vi "GUI_Beampointing2.vi"() -> ()   [LabVIEW 2011]
uses:
  GUI_Template/GUI_master/tcp_new_data_event.ctl
  GUI_Template/GUI_master/tcp new data cluster.ctl
  Device Driver/TRAServer/StatusTRA_TypDef.ctl
  Ctrs/beam detection.ctl
  Ctrs/move.ctl
  Ctrs/stats.ctl
  <vilib>/Analysis/NI_AALBase.lvlib
  Device Driver/TRAServer/TRAServer.lvclass
panel:
  in  "Set Centriod Target":bool
  in  "size":dbl=68.1
  in  "Tab Control 2":enum32{"CCD Original ", "CCD Detected"}(tab)=enum."CCD Detected"
  out "image::1":T1(plugin-control) caption="StagingM1Far"
  out "Beam":T1(plugin-control)
  in  "Reset History":bool
  out "centriod X":dbl[](graph)=[269.2727355957031, 269.2727355957031, 269.3190002441406]
  out "centriod Y":dbl[](graph)=[287.58294677734375, 287.58294677734375, 287.771484375]
  out "Stats":cluster{timestamp[], dbl[]}[](graph)
  out "move.Stepsize 2":dbl
  out "move.Stepsize":dbl
  in  "Tab Control":enum32{"System", "Detection", "Feedback"}(tab)=enum."Detection"
  in  "Save Stats":bool
  in  "update speed [ms]":i32=100
  in  "img to avg":i32=5
  in  "Save Config":bool
  in  "Load Config":bool
  in  "UDP Error Message":string
  in  "Cameras":u16(ring)=15 items=["10TW_Driver_Spot_Cam", "B1_TelInput", "B5_CompOut", "B6_SwitchYNear", "GIGEtest", "L7_TREXPass4", "L8_M10Leak", "OAPtestCam", "PaperCam", "StagingAlignBeam1", "StagingAlignBeam2", "StagingCapAlignment", "StagingCapSpec", "StagingCapSpec1stOrder", "StagingChromaxGuppy", "StagingDiodeMonitor", "StagingFocusBeam1", "StagingFocusBeam2", "StagingGuppy", "StagingM1Far", "StagingM1Near", "StagingM3Far", "StagingM4", "StagingM5", "StagingMagnetCam1", "StagingMagnetCam2", "StagingMagnetCam3", "StagingManta2", "StagingModeImager2", "StagingModeTemp", "StagingOAP1Far", "StagingOAP1Near", "StagingOAP2Far", "StagingOAP2Near", "StagingPhasics", "StagingPhosphor", "StagingTapeCam", "StagingTapeMonitorCam", "TREXVarianCam0", "TREXVarianCam1", "TREXVarianCam2", "TREXVarianCam3", "TREX_CapSideView", "TREX_TA6", "TS-253a_in", "TS-CapSideview", "TS-CapSpec", "TS-ChromexCam", "TS-InputNearField", "TS-Mode1", "TS-OverlapCam", "TS-Periscope", "XUV_Cam1", "XUV_Cam2"]
  in  "beam detection para":T2={"Filter"=1, "Filter Para"={"X Size"=5, "Y Size"=5, "% Tolerance"=1}, "detection method"=4, "smal para"=[{"Measurement Parameter"=35, "Range Lower Value"=0.0, "Range Upper Value"=500.0, "Range"=TRUE, "Measurement Type"=FALSE}], "Remove small Objects"=TRUE, "Restrict to round Objects"=TRUE} {"smal para"."Measurement Parameter" items=["Center of Mass X", "Center of Mass Y", "First Pixel X", "First Pixel Y", "Bounding Rect Left", "Bounding Rect Top", "Bounding Rect Right", "Bounding Rect Bottom", "Max Feret Diameter Start X", "Max Feret Diameter Start Y", "Max Feret Diameter End X", "Max Feret Diameter End Y", "Max Horiz. Segment Length Left", "Max Horiz. Segment Length Right", "Max Horiz. Segment Length Row", "-", "Bounding Rect Width", "Bounding Rect Height", "Bounding Rect Diagonal", "Perimeter", "Convex Hull Perimeter", "Holes' Perimeter", "Max Feret Diameter", "Equivalent Ellipse Major Axis", "Equivalent Ellipse Minor Axis", "Equivalent Ellipse Minor Axis (Feret)", "Equivalent Rect Long Side", "Equivalent Rect Short Side", "Equivalent Rect Diagonal", "Equivalent Rect Short Side (Feret)", "Average Horiz. Segment Length", "Average Vert. Segment Length", "Hydraulic Radius", "Waddel Disk Diameter", "-", "Area", "Holes' Area", "Particle & Holes' Area", "Convex Hull Area", "Image Area", "-", "Number of Holes", "Number of Horiz. Segments", "Number of Vert. Segments", "-", "Orientation", "Max Feret Diameter Orientation", "-", "% Area/Image Area", "% Area/(Particle & Holes' Area)", "Ratio of Equivalent Ellipse Axes", "Ratio of Equivalent Rect Sides", "-", "Elongation Factor", "Compactness Factor", "Heywood Circularity Factor", "Type Factor", "-", "Sum X", "Sum Y", "Sum XX", "Sum XY", "Sum YY", "Sum XXX", "Sum XXY", "Sum XYY", "Sum YYY", "-", "Moment of Inertia XX", "Moment of Inertia XY", "Moment of Inertia YY", "Moment of Inertia XXX", "Moment of Inertia XXY", "Moment of Inertia XYY", "Moment of Inertia YYY", "Norm. Moment of Inertia XX", "Norm. Moment of Inertia XY", "Norm. Moment of Inertia YY", "Norm. Moment of Inertia XXX", "Norm. Moment of Inertia XXY", "Norm. Moment of Inertia XYY", "Norm. Moment of Inertia YYY", "Hu Moment 1", "Hu Moment 2", "Hu Moment 3", "Hu Moment 4", "Hu Moment 5", "Hu Moment 6", "Hu Moment 7"]; "smal para"."Range Lower Value" format="%.2f"; "smal para"."Range Upper Value" format="%.2f"; "detection method" items=["clustering", "entropy", "metric", "moments", "inter-class variance"]; "Filter" items=["No Filter", "Median Filter", "Low Pass Filter"]}
  in  "Move Properties":T4={"Tolerance [%]"=10.0, "Stepsize"=0.0, "Invert Axis"=FALSE, "Invert Direction X"=FALSE, "Invert Direction Y"=FALSE, "enable feedback"=FALSE} {"Stepsize" format="%#_6p"}
  out "Y Size":dbl=130.0
  out "X Size":dbl=136.2
  out "Particle Reports (Pixels)":T5(array[cluster])=[{"Area"=12832.0, "Number of Holes"=0.0, "Bounding Rect"={"Left"=200.0, "Top"=223.0, "Right"=335.0, "Bottom"=353.0}, "Center of Mass"={"X"=268.7340243142145, "Y"=287.8902743142145}, "Orientation"=19.894021936277838, "Dimensions"={"Width"=135.0, "Height"=130.0}}] {"Orientation" format="%.2f"; "Dimensions"."Height" format="%.2f"; "Dimensions"."Width" format="%.2f"; "Center of Mass"."Y" format="%.2f"; "Center of Mass"."X" format="%.2f"; "Bounding Rect"."Bottom" format="%.2f"; "Bounding Rect"."Right" format="%.2f"; "Bounding Rect"."Top" format="%.2f"; "Bounding Rect"."Left" format="%.2f"; "Number of Holes" format="%.2f"; "Area" format="%.2f"}
  in  "save cluster":T6={"img to avg"=0, "beam detection para"={"Filter"=0, "Filter Para"={"X Size"=0, "Y Size"=0, "% Tolerance"=0}, "detection method"=0, "smal para"=[], "Remove small Objects"=FALSE, "Restrict to round Objects"=TRUE}, "move"={"Tolerance [%]"=0.0, "Stepsize"=0.0, "Invert Axis"=FALSE, "Invert Direction X"=FALSE, "Invert Direction Y"=FALSE, "enable feedback"=FALSE}} {"beam detection para"."smal para"."Measurement Parameter" items=["Center of Mass X", "Center of Mass Y", "First Pixel X", "First Pixel Y", "Bounding Rect Left", "Bounding Rect Top", "Bounding Rect Right", "Bounding Rect Bottom", "Max Feret Diameter Start X", "Max Feret Diameter Start Y", "Max Feret Diameter End X", "Max Feret Diameter End Y", "Max Horiz. Segment Length Left", "Max Horiz. Segment Length Right", "Max Horiz. Segment Length Row", "-", "Bounding Rect Width", "Bounding Rect Height", "Bounding Rect Diagonal", "Perimeter", "Convex Hull Perimeter", "Holes' Perimeter", "Max Feret Diameter", "Equivalent Ellipse Major Axis", "Equivalent Ellipse Minor Axis", "Equivalent Ellipse Minor Axis (Feret)", "Equivalent Rect Long Side", "Equivalent Rect Short Side", "Equivalent Rect Diagonal", "Equivalent Rect Short Side (Feret)", "Average Horiz. Segment Length", "Average Vert. Segment Length", "Hydraulic Radius", "Waddel Disk Diameter", "-", "Area", "Holes' Area", "Particle & Holes' Area", "Convex Hull Area", "Image Area", "-", "Number of Holes", "Number of Horiz. Segments", "Number of Vert. Segments", "-", "Orientation", "Max Feret Diameter Orientation", "-", "% Area/Image Area", "% Area/(Particle & Holes' Area)", "Ratio of Equivalent Ellipse Axes", "Ratio of Equivalent Rect Sides", "-", "Elongation Factor", "Compactness Factor", "Heywood Circularity Factor", "Type Factor", "-", "Sum X", "Sum Y", "Sum XX", "Sum XY", "Sum YY", "Sum XXX", "Sum XXY", "Sum XYY", "Sum YYY", "-", "Moment of Inertia XX", "Moment of Inertia XY", "Moment of Inertia YY", "Moment of Inertia XXX", "Moment of Inertia XXY", "Moment of Inertia XYY", "Moment of Inertia YYY", "Norm. Moment of Inertia XX", "Norm. Moment of Inertia XY", "Norm. Moment of Inertia YY", "Norm. Moment of Inertia XXX", "Norm. Moment of Inertia XXY", "Norm. Moment of Inertia XYY", "Norm. Moment of Inertia YYY", "Hu Moment 1", "Hu Moment 2", "Hu Moment 3", "Hu Moment 4", "Hu Moment 5", "Hu Moment 6", "Hu Moment 7"]; "beam detection para"."smal para"."Range Lower Value" format="%.2f"; "beam detection para"."smal para"."Range Upper Value" format="%.2f"; "beam detection para"."detection method" items=["clustering", "entropy", "metric", "moments", "inter-class variance"]; "beam detection para"."Filter" items=["No Filter", "Median Filter", "Low Pass Filter"]}
  out "move required":bool
  out "moving":bool
  out "Best Rectangle":T7(array[cluster])=[{"Left"=200.0, "Top"=223.0, "Right"=338.0, "Bottom"=353.0}, {"Left"=200.0, "Top"=223.0, "Right"=338.0, "Bottom"=353.0}, {"Left"=205.0, "Top"=224.0, "Right"=338.0, "Bottom"=350.0}, {"Left"=200.0, "Top"=223.0, "Right"=336.0, "Bottom"=355.0}, {"Left"=200.0, "Top"=223.0, "Right"=336.0, "Bottom"=355.0}]
  out "XY Graph":cluster{timestamp[], dbl[]}[](graph)=[{[timestamp(3452404798.8513913 s since 1904-01-01), timestamp(3452404799.6214356 s since 1904-01-01), timestamp(3452404800.2504716 s since 1904-01-01), timestamp(3452404800.877507 s since 1904-01-01), timestamp(3452404801.5115438 s since 1904-01-01), timestamp(3452404802.1385794 s since 1904-01-01), timestamp(3452404802.7796164 s since 1904-01-01), timestamp(3452404803.4086523 s since 1904-01-01), timestamp(3452404804.1166925 s since 1904-01-01), timestamp(3452404804.7627296 s since 1904-01-01), timestamp(3452404805.403766 s since 1904-01-01), timestamp(3452404806.046803 s since 1904-01-01), timestamp(3452404806.8958516 s since 1904-01-01), timestamp(3452404807.531888 s since 1904-01-01), timestamp(3452404808.174925 s since 1904-01-01), timestamp(3452404808.811961 s since 1904-01-01), timestamp(3452404809.4529977 s since 1904-01-01), timestamp(3452404810.0910344 s since 1904-01-01), timestamp(3452404810.732071 s since 1904-01-01), timestamp(3452404811.373108 s since 1904-01-01)], [-3.53924560546875, -4.652754657642788, -5.44743290091867, -5.300940785876151, -4.715238659785825, -6.004101011596333, -4.752166041728003, -5.050226506875958, -4.109178710453193, -4.665509033203136, -5.175085449218727, -5.028265380859352, -4.379766845703102, -4.631829833984398, -4.844409179687489, -4.304394531250011, -4.530322265624989, -4.936749267578136, -4.763983154296852, -4.448400878906227]}, {[timestamp(3452404798.8513913 s since 1904-01-01), timestamp(3452404799.6214356 s since 1904-01-01), timestamp(3452404800.2504716 s since 1904-01-01), timestamp(3452404800.877507 s since 1904-01-01), timestamp(3452404801.5115438 s since 1904-01-01), timestamp(3452404802.1385794 s since 1904-01-01), timestamp(3452404802.7796164 s since 1904-01-01), timestamp(3452404803.4086523 s since 1904-01-01), timestamp(3452404804.1166925 s since 1904-01-01), timestamp(3452404804.7627296 s since 1904-01-01), timestamp(3452404805.403766 s since 1904-01-01), timestamp(3452404806.046803 s since 1904-01-01), timestamp(3452404806.8958516 s since 1904-01-01), timestamp(3452404807.531888 s since 1904-01-01), timestamp(3452404808.174925 s since 1904-01-01), timestamp(3452404808.811961 s since 1904-01-01), timestamp(3452404809.4529977 s since 1904-01-01), timestamp(3452404810.0910344 s since 1904-01-01), timestamp(3452404810.732071 s since 1904-01-01), timestamp(3452404811.373108 s since 1904-01-01)], [1.230804443359375, -0.3328436558336989, 0.6609996983648898, -0.3690822614664171, 0.27569034847687135, -0.11031780080207909, -0.31644478020683664, 0.5764054032015906, 0.6783385802021371, 0.532257080078125, 0.9677673339843977, 0.27269287109373863, 0.38755493164063637, 0.46185302734375, 0.137542724609375, 0.073089599609375, 0.6028076171875227, 0.7097961425781136, 1.0255981445312727, 0.9409057617187386]}]
  out "Y offset":dbl=0.9409057617187386
  out "X offset":dbl=-4.448400878906227
  in  "Target.X::1":dbl=265.0 min=0.0 max=2000.0 format="%#_6f"
  in  "Target.Y::1":dbl=288.0 min=0.0 max=2000.0 format="%#_6f"
  out "mean Y":dbl=287.05909423828126 format="%0.2f"
  out "mean X":dbl=269.4484008789062 format="%0.2f"
  out "beam detected":bool=TRUE
  in  "Status.Axis 2::2":T8=enum."DISABLE" caption="Status.Axis 1::2"
  in  "Status.Axis 1::2":T8=enum."DISABLE"
  in  "Position.Axis 1::2":dbl=1.39334 caption="TREX M20 X" min=0.0 max=6.0 format="%#_6f"
  in  "Position.Axis 2::2":dbl=4.66198 caption="TREX M20 Y" min=0.0 max=7.0 format="%#_6f"
  in  "GUIdevice 2":string="TREX TRA1"
  out "error out":errorcluster
  in  "insert tag":bool=TRUE
  in  "stop":bool=TRUE
  in  "GUIdevice 1":string="PaperCam"
  out "tcp data event":T9
  out "error IO 2":errorcluster
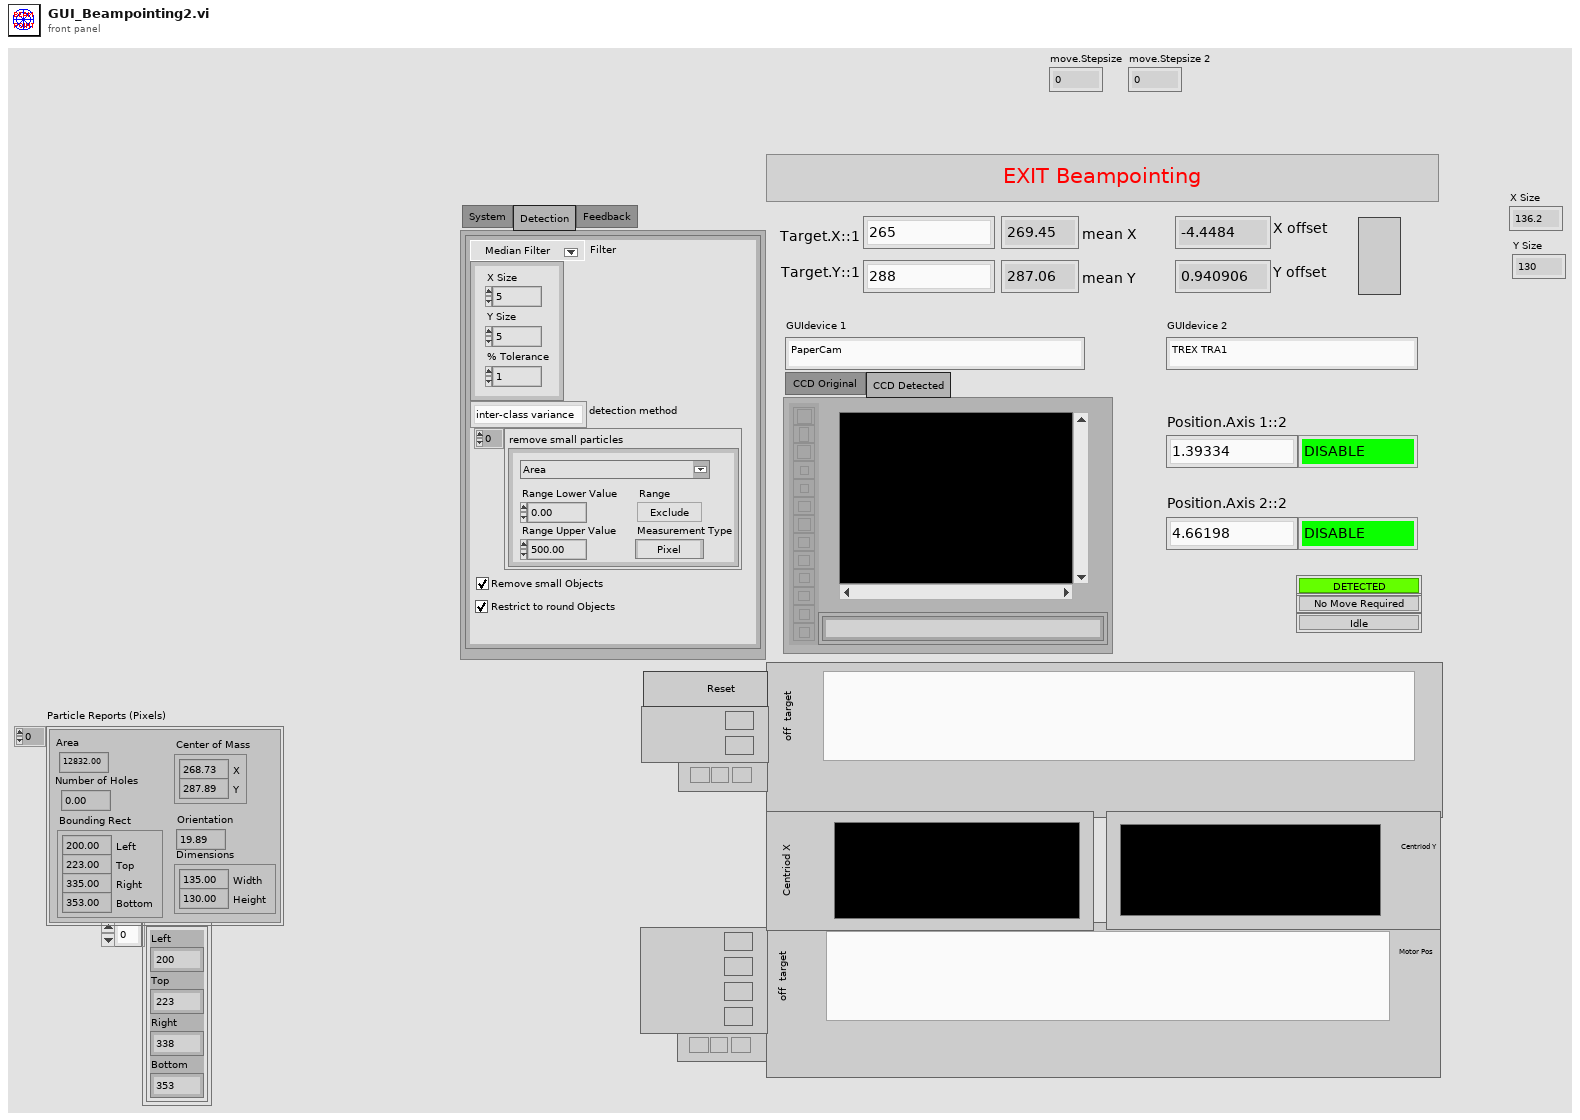
[diagram p1: front panel]
types:
  T1 = typedef "IMAQ Image.ctl" = refnum<image>
  T2 = typedef "beam detection.ctl" = cluster{"Filter":u16, "Filter Para":cluster{"X Size":i32, "Y Size":i32, "% Tolerance":i32}, "detection method":i32, "smal para":cluster{"Measurement Parameter":T3, "Range Lower Value":dbl, "Range Upper Value":dbl, "Range":bool, "Measurement Type":bool}[], "Remove small Objects":bool, "Restrict to round Objects":bool}
  T3 = typedef "Particle Parameters" = i32
  T4 = typedef "move.ctl" = cluster{"Tolerance [%]":dbl, "Stepsize":dbl, "Invert Axis":bool, "Invert Direction X":bool, "Invert Direction Y":bool, "enable feedback":bool}
  T5 = cluster{"Area":dbl, "Number of Holes":dbl, "Bounding Rect":cluster{"Left":dbl, "Top":dbl, "Right":dbl, "Bottom":dbl}, "Center of Mass":cluster{"X":dbl, "Y":dbl}, "Orientation":dbl, "Dimensions":cluster{"Width":dbl, "Height":dbl}}[]
  T6 = cluster{"img to avg":i32, "beam detection para":T2, "move":T4}
  T7 = cluster{"Left":dbl, "Top":dbl, "Right":dbl, "Bottom":dbl}[]
  T8 = typedef "TRAServer.lvclass/StatusTRA_TypDef.ctl" = enum16{"NOT REFERENCED", "CONFIGURATION", "HOMING", "MOVING", "READY", "DISABLE", "JOGGING"}
  T9 = typedef "tcp_new_data_event.ctl" = refnum<user-event>
  T10 = typedef "tcp new data cluster.ctl" = cluster{"EventEnum":enum16{"new data", "connection status update"}, "Device name":string}
  T11 = typedef "Image Type" = u32
  T12 = cluster{"Left":i32, "Top":i32, "Right":i32, "Bottom":i32}
  T13 = enum32{"invalid app kind", "Development System", "Run Time System", "Student Edition", "Embedded LabVIEW", "Evaluation", "Custom"}
  T14 = enum32{"Invalid", "Standard", "Closed", "Hidden", "Minimized", "Maximized"}
  T15 = enum16{"open", "replace", "create", "open or create", "replace or create", "replace or create with confirmation"}
  T16 = typedef "stats.ctl" = cluster{"Stat Centriod X":dbl[], "Stat Centriod Y":dbl[], "TRA Position X":dbl[], "TRA PositionY":dbl[], "Time":timestamp[]}
  T17 = cluster{"Core":cluster{"Current VI Reference":refnum<vi>, "Close Panel on Exit?":bool}, "beam detection para":T2, "Centriod X":dbl[], "Centriod Y":dbl[], "Best Rectangle":cluster{"Left":dbl, "Top":dbl, "Right":dbl, "Bottom":dbl}[], "PArticle Report":cluster{"Area":dbl, "Number of Holes":dbl, "Bounding Rect":cluster{"Left":dbl, "Top":dbl, "Right":dbl, "Bottom":dbl}, "Center of Mass":cluster{"X":dbl, "Y":dbl}, "Orientation":dbl, "Dimensions":cluster{"Width":dbl, "Height":dbl}}[], "Mean Centriod X":dbl[], "Mean Centriod Y":dbl[], "Time":timestamp[], "beam detected":bool, "offsets":cluster{"X offset":dbl, "Y offset":dbl}, "move":T4, "moving":bool, "Stats":T16, "set centriod target":bool}
  T18 = cluster{"Left":dbl, "Top":dbl, "Right":dbl, "Bottom":dbl}
  T19 = cluster{"Current VI Reference":refnum<vi>, "Close Panel on Exit?":bool}
  T20 = cluster{"Time":timestamp[], "Stat Centriod X":dbl[]}
  T21 = cluster{"Time":timestamp[], "Stat Centriod Y":dbl[]}
  T22 = cluster{"Time":timestamp[], "TRA Position X":dbl[]}
  T23 = cluster{"Time":timestamp[], "TRA PositionY":dbl[]}
  T24 = cluster{"Time":timestamp[], "TRA PositionY":dbl[]}[]
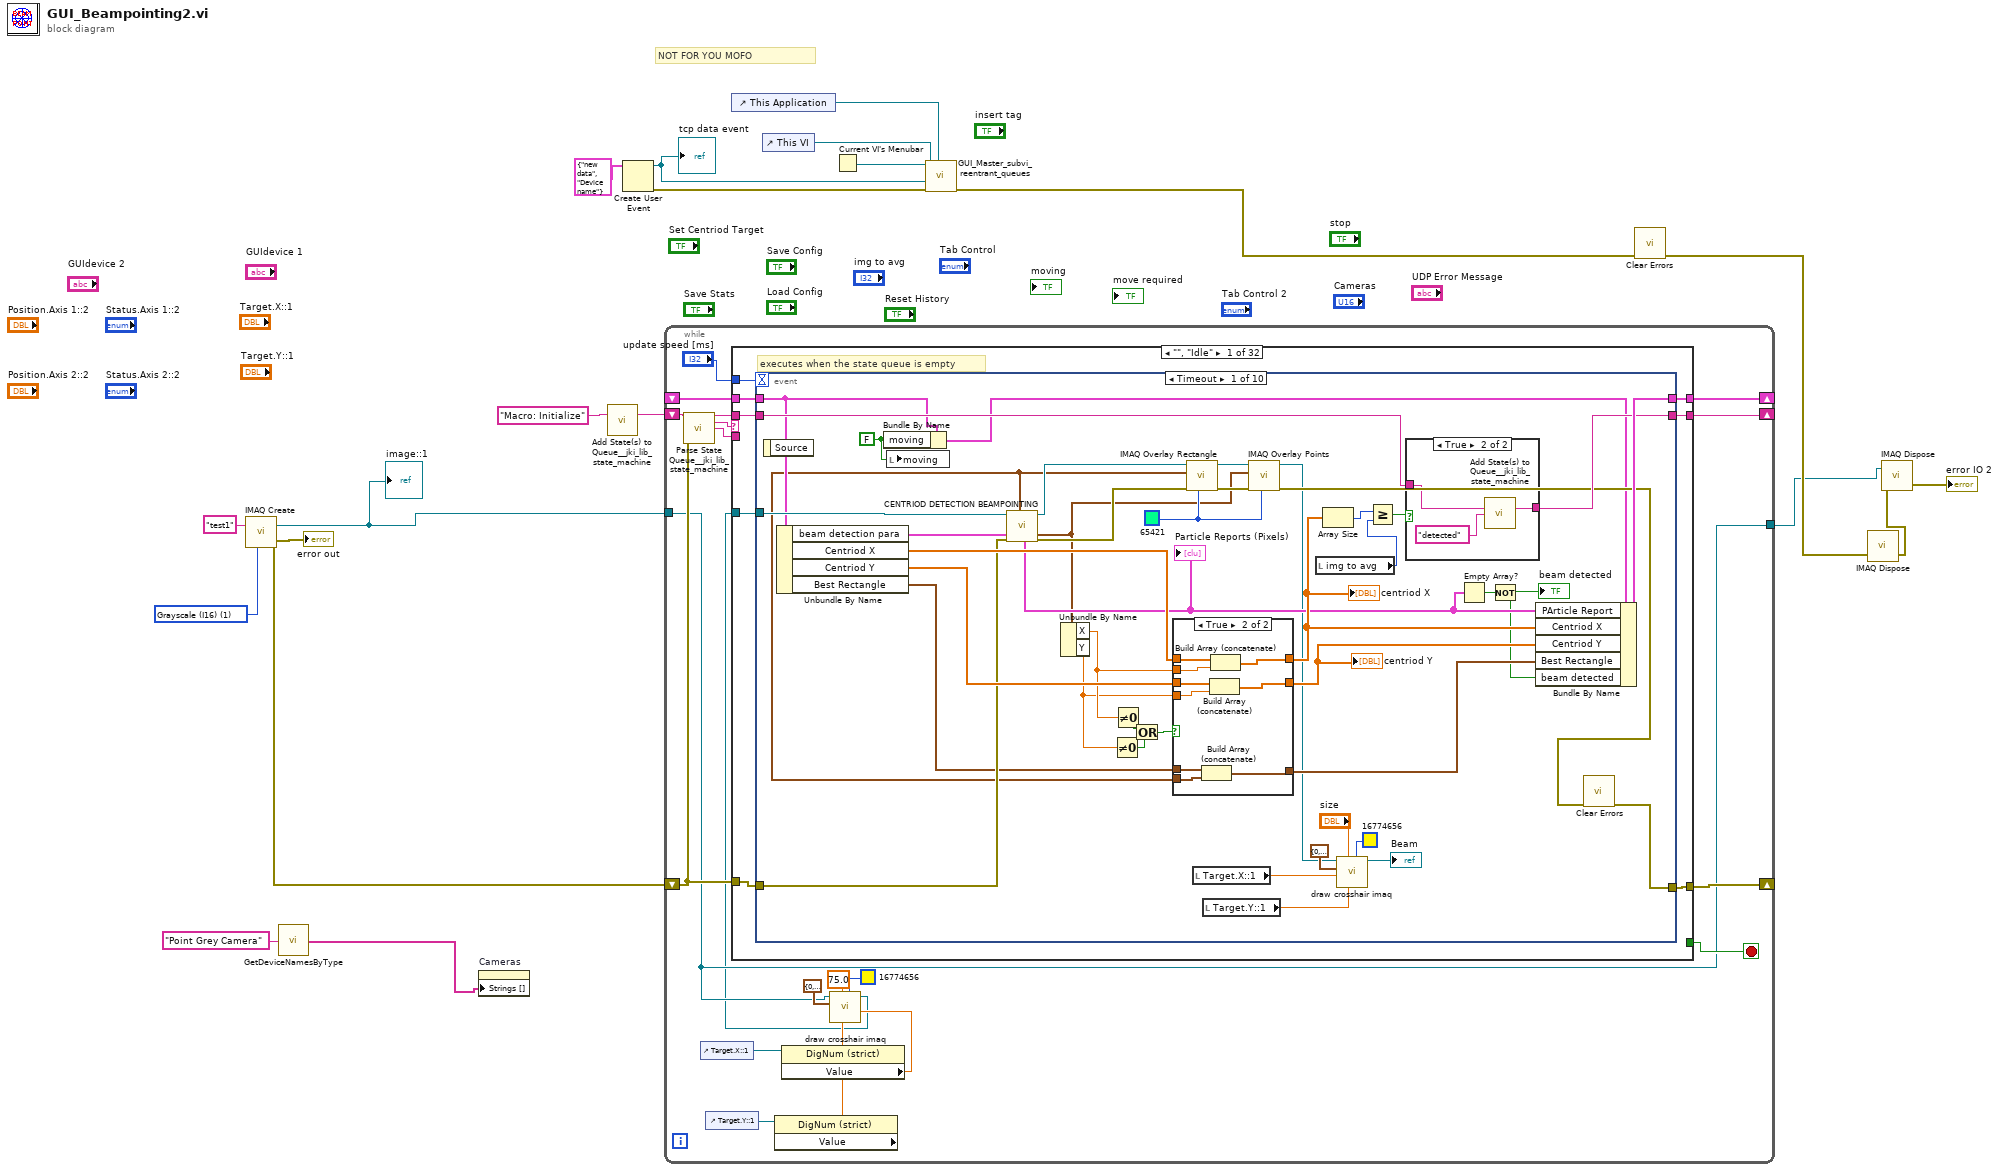
[diagram p0: block diagram]
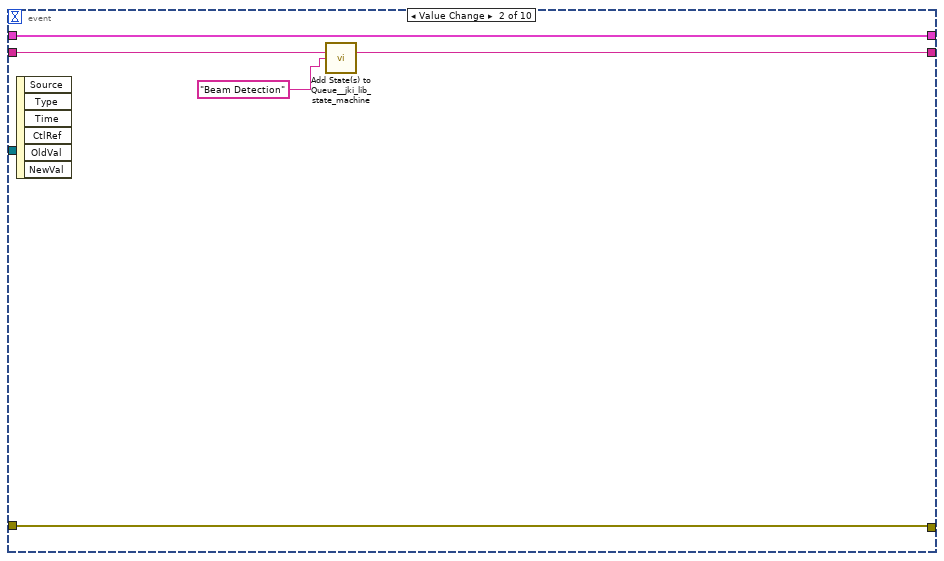
[diagram p4: hidden frame]
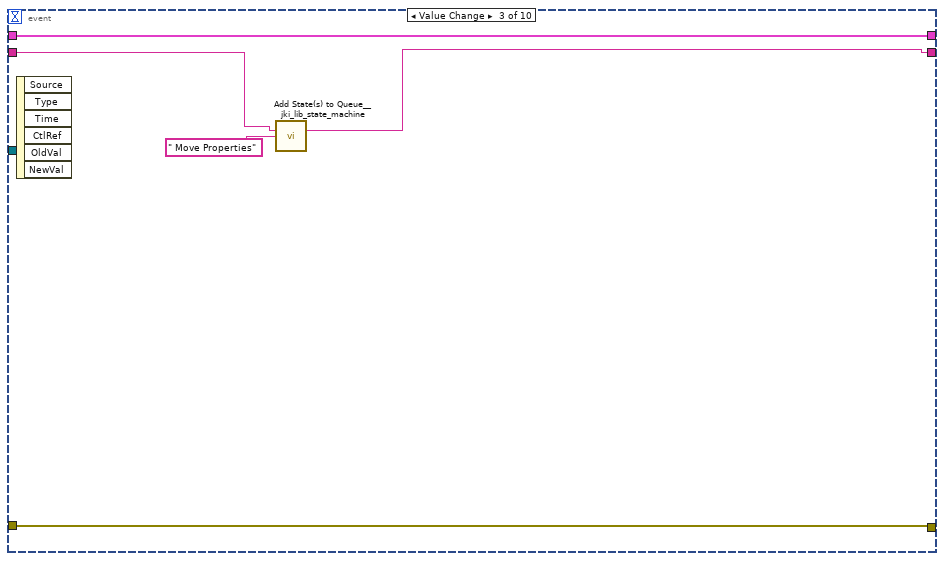
[diagram p5: hidden frame]
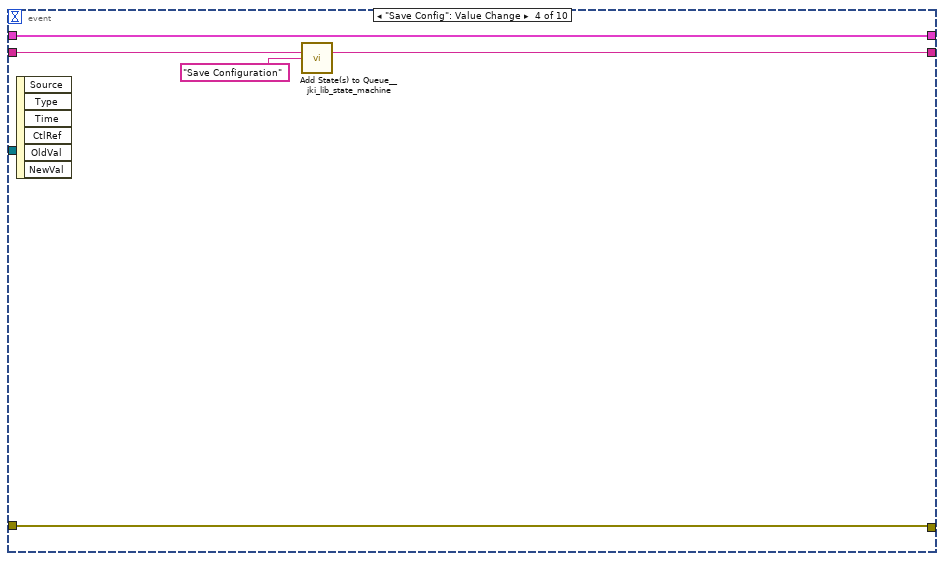
[diagram p6: hidden frame]
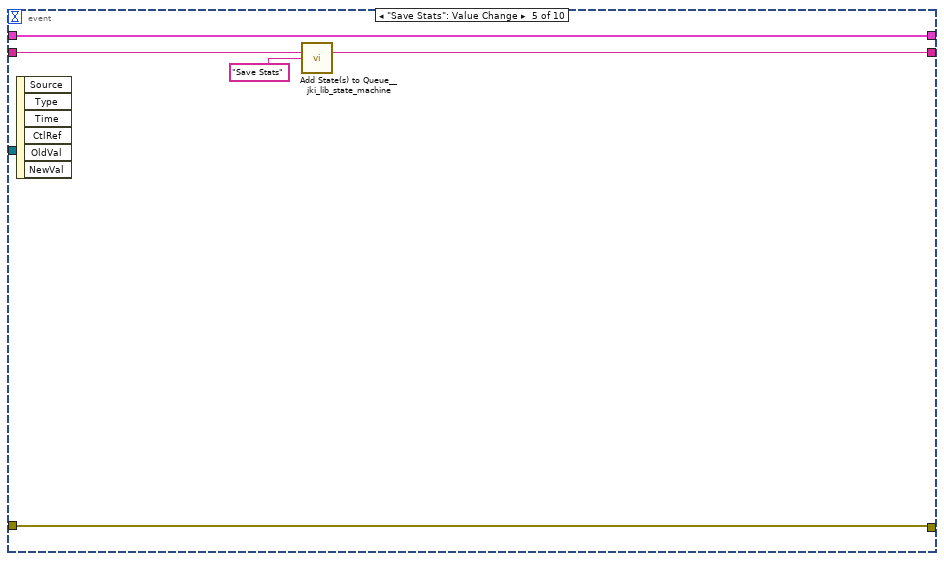
[diagram p7: hidden frame]
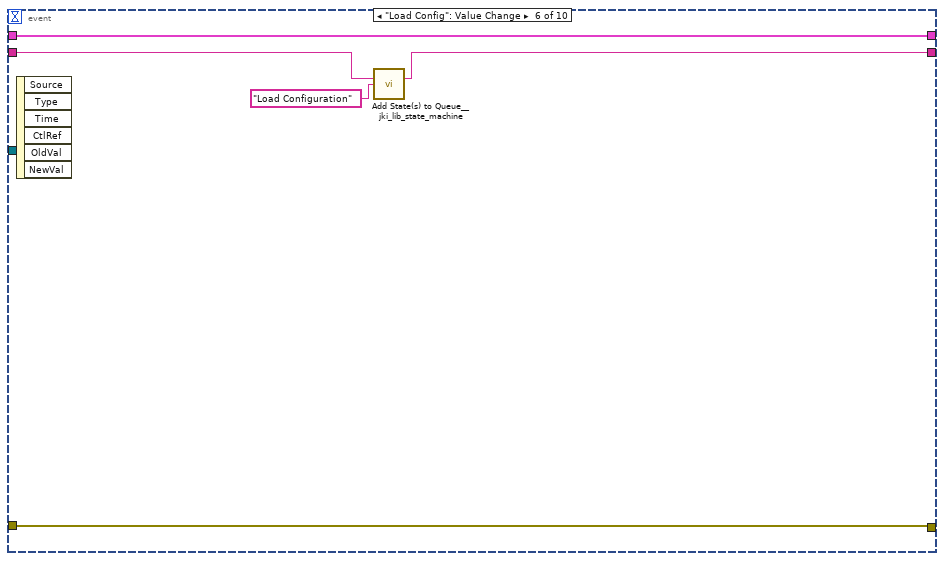
[diagram p8: hidden frame]
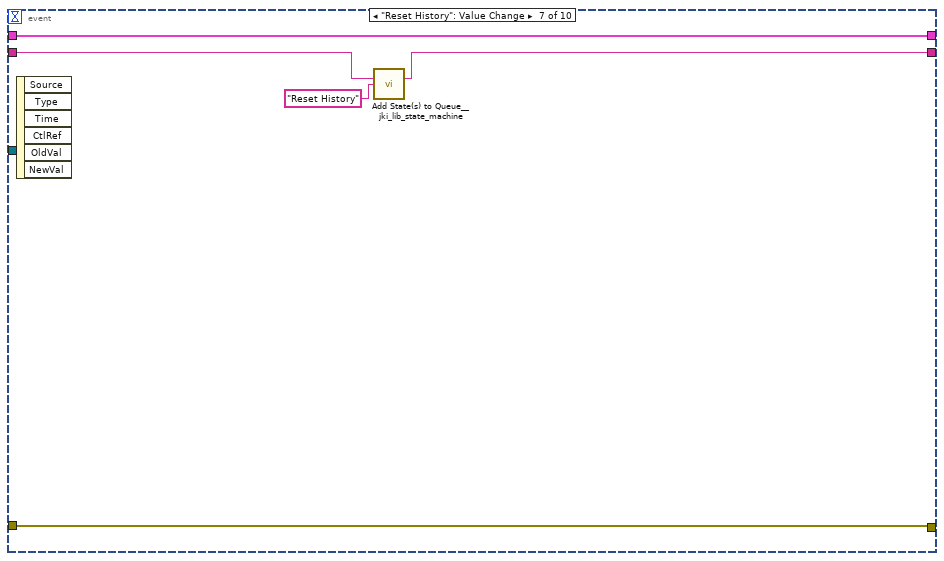
[diagram p9: hidden frame]
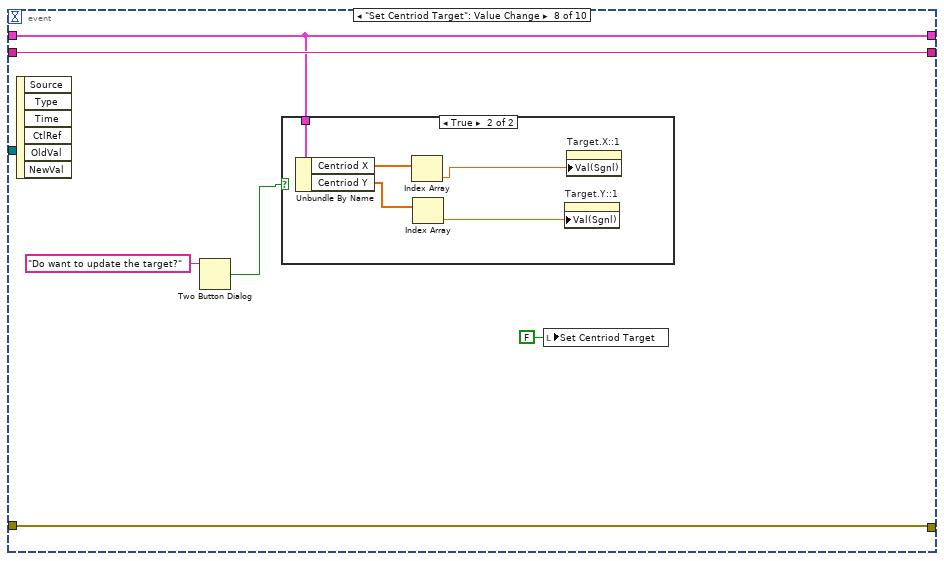
[diagram p10: hidden frame]
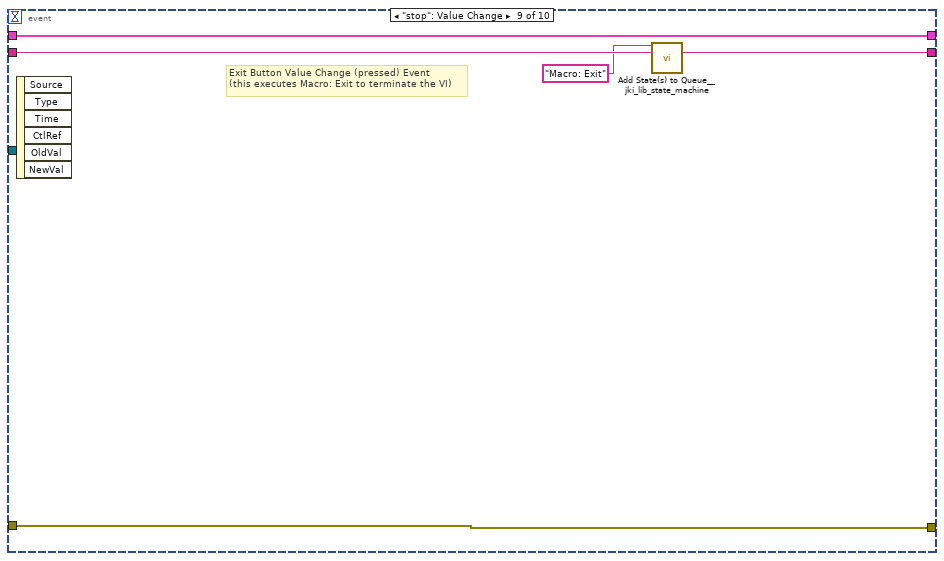
[diagram p12: hidden frame]
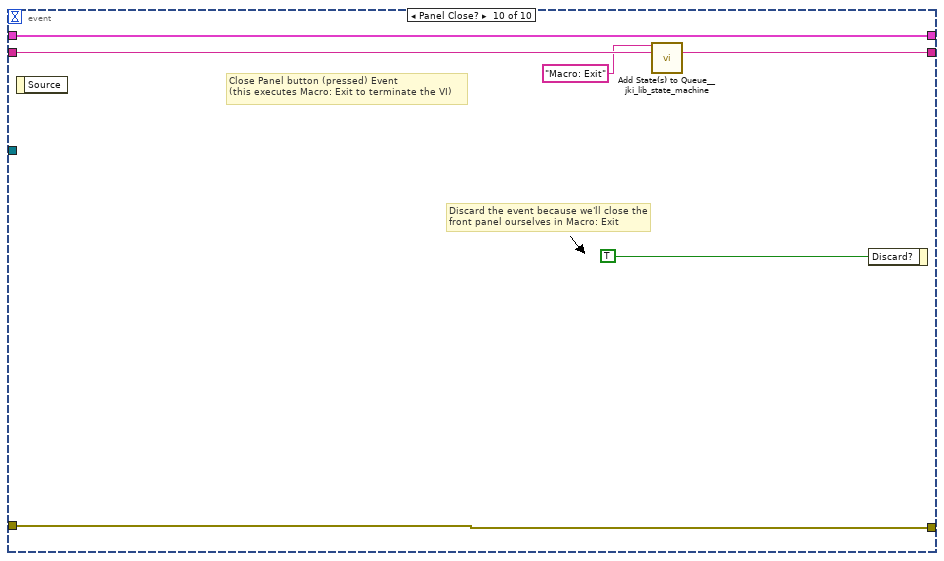
[diagram p13: hidden frame]
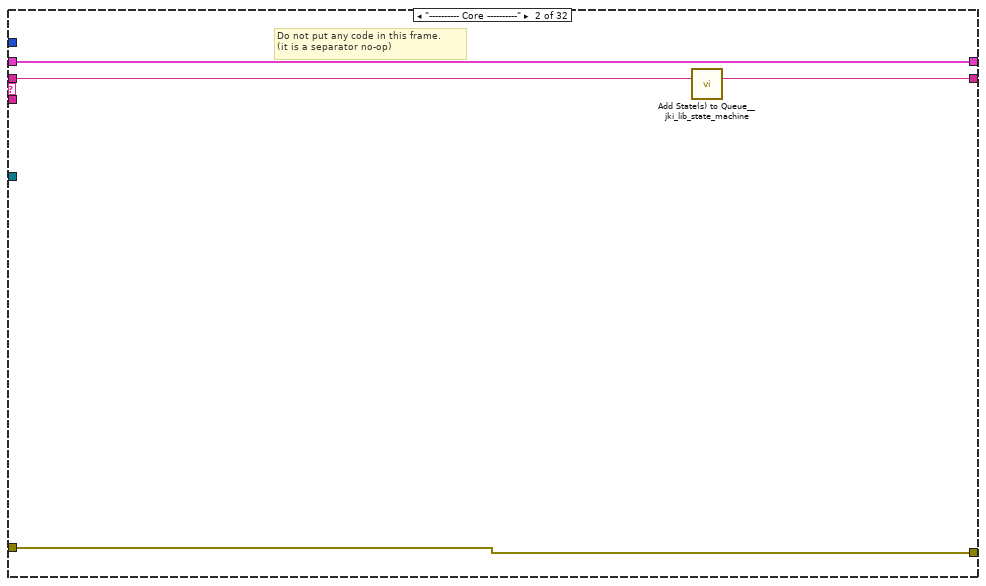
[diagram p14: hidden frame]
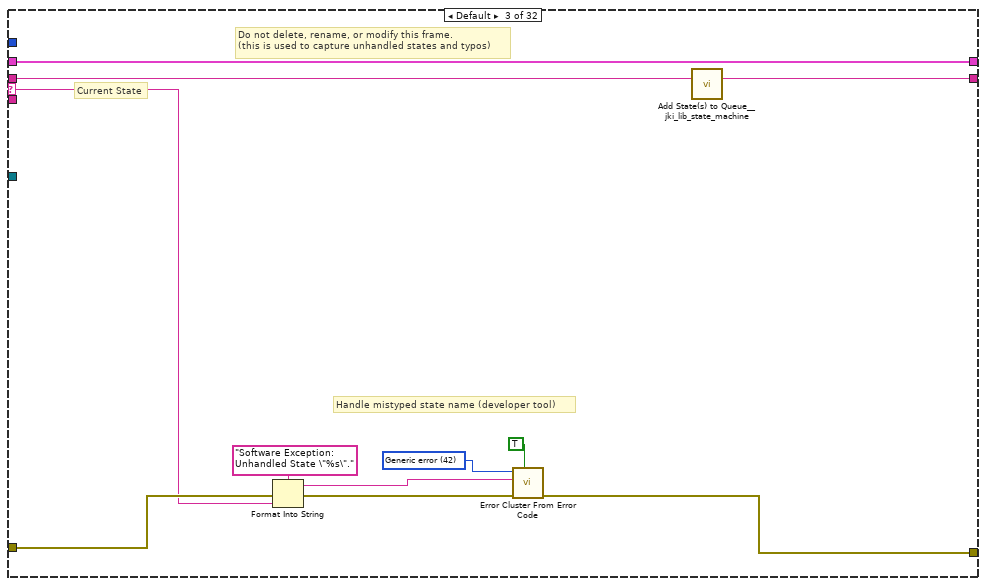
[diagram p15: hidden frame]
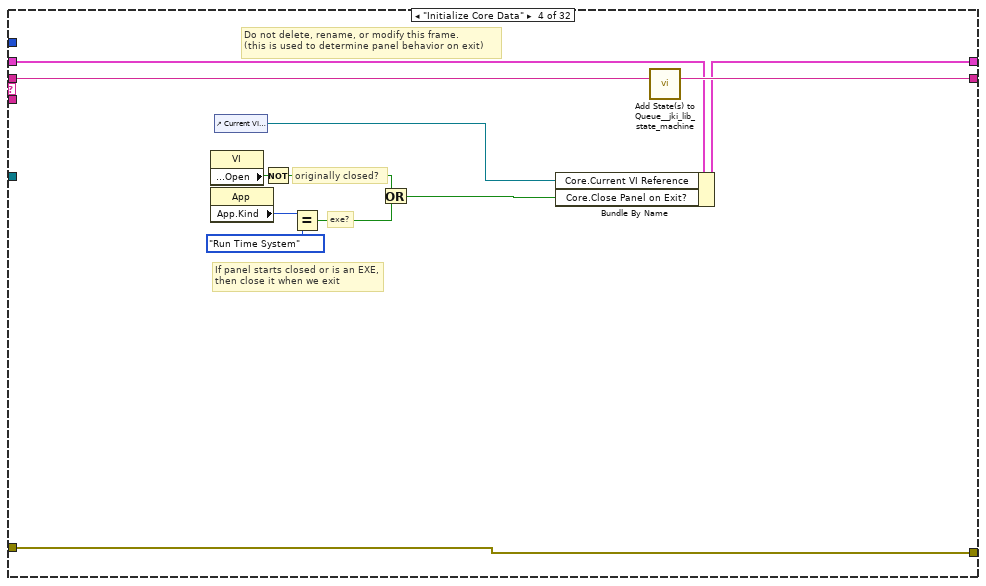
[diagram p16: hidden frame]
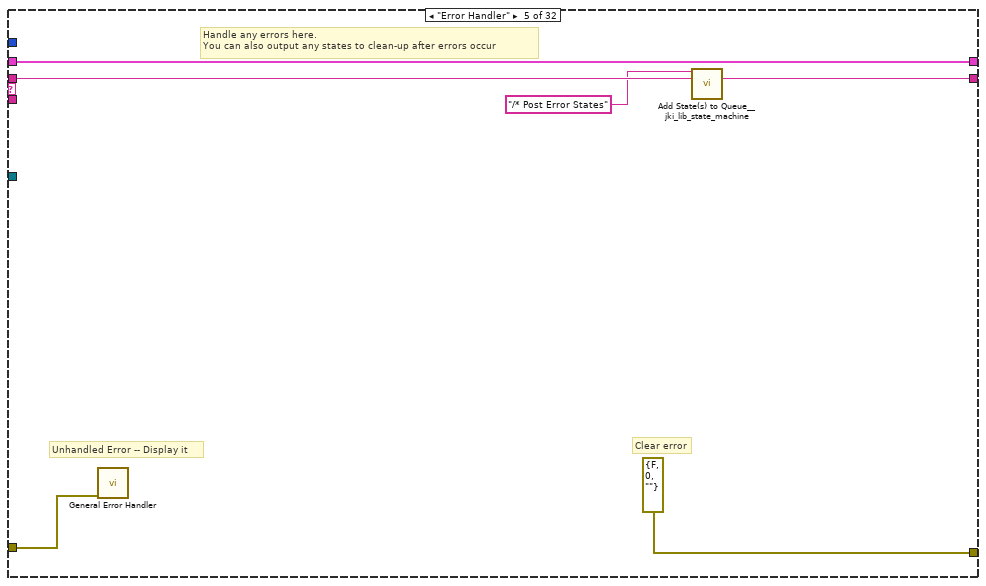
[diagram p17: hidden frame]
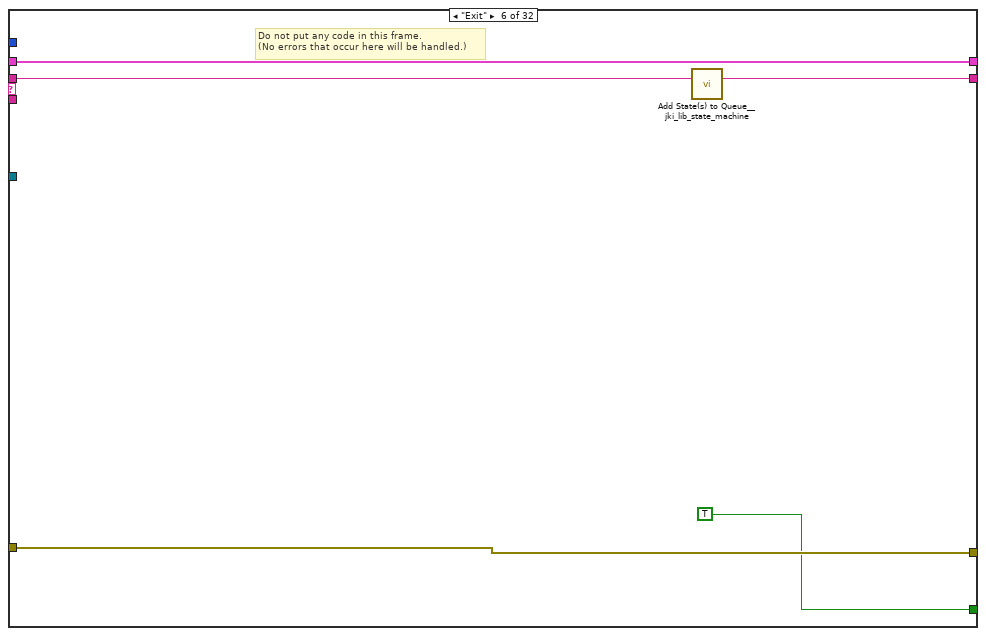
[diagram p18: hidden frame]
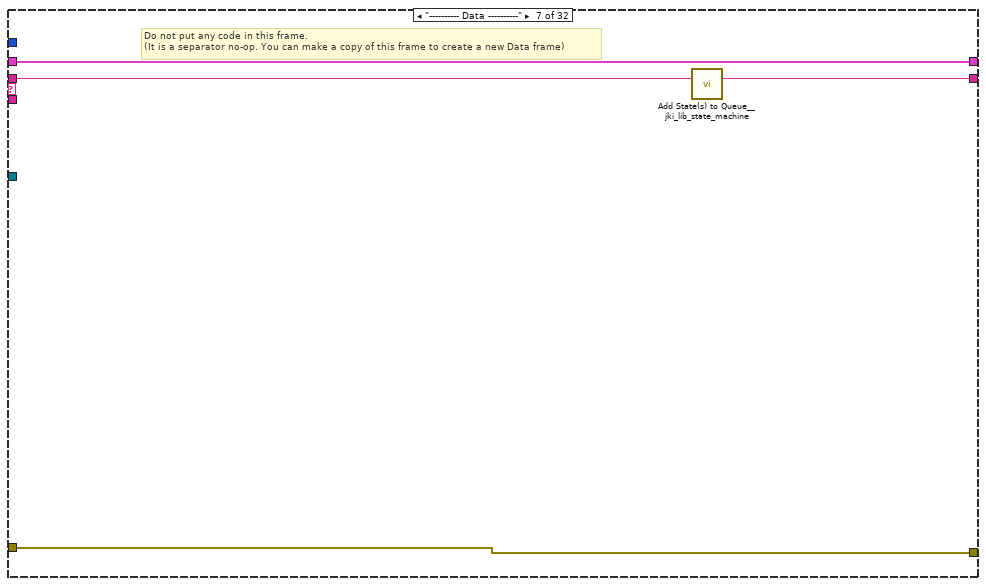
[diagram p19: hidden frame]
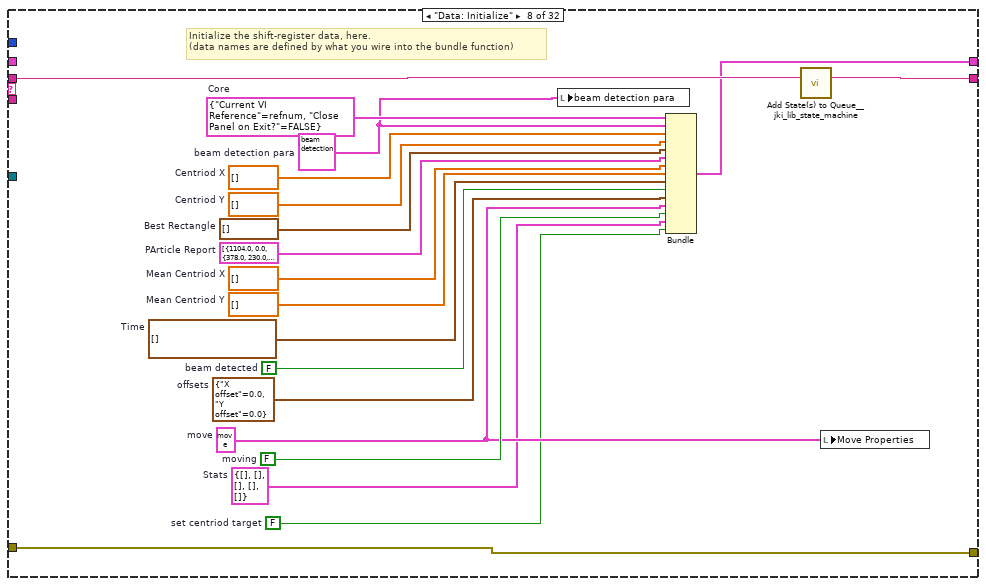
[diagram p20: hidden frame]
diagram:
  w18 = T11 1 items=["Grayscale (U8)", "Grayscale (I16)", "Grayscale (SGL)", "Complex (CSG)", "RGB (U32)", "HSL (U32)", "RGB (U64)", "Grayscale (U16)"] ("Image Type")
  # "NOT FOR YOU MOFO"
  n1 = call "IMAQ Create"("Image Name"="test1", "Image Type"=w18) -> ("New Image"=w3:T1, "error out"=w11:errorcluster)  [unwired: 3 in]
  "error out" <- w11
  "image::1" <- w3
  n2 = call "GetDeviceNamesByType.vi"("Device Type"="Point Grey Camera") -> ("Array"=w1:string[])
  n3 = property on="Cameras" class="Ring (strict)"("Strings []"=w1) -> ()  [unwired: 2 in, 2 out]
  n4 = call <vilib>:"Add State(s) to Queue__jki_lib_state_machine.vi"("State(s) in (\"\")"="Macro: Initialize") -> ("States Out"=w13:string)  [unwired: 14 in]
  n5 = Create User Event(user event datatype=T10 {"EventEnum"=enum."new data", "Device name"="Device name"} ("New Event")) -> (user event=w4:refnum<user-event>, error out=w6:errorcluster)  [unwired: 1 in]
  "tcp data event" <- w4
  n6 = while "JKI - String-Based Queued State Machine (Basic) v1.0" {
    shift-right: [w33] -> _
    shift-left: _ -> [w32]
    shift-right: [w35] -> _
    shift-left: w11 -> [w30]
    shift-right: [w34] -> _
    shift-left: w13 -> [w36]
    tunnel: w3 -> [w21]
    tunnel: [w21] -> w10
    stop <- w29 stop-if-true
    n7 = call <vilib>:"Parse State Queue__jki_lib_state_machine.vi"("State Queue"=w36, "Error In (no error)"=w30) -> ("Remaining States"=w38:string, "Current State"=w39:string, "Arguments"=w37:string)  [unwired: 11 in]
    n8 = control-ref of="Target.X::1"() -> (w25:refnum<vi>)
    n9 = control-ref of="Target.Y::1"() -> (w26:refnum<vi>)
    n10 = property class="DigNum (strict)"(reference=w26) -> ("Value"=w28:dbl)  [unwired: 1 in, 2 out]
    n11 = property class="DigNum (strict)"(reference=w25) -> ("Value"=w27:dbl)  [unwired: 1 in, 2 out]
    n12 = call "draw crosshair imaq.vi"("Color"=u32 16774656, "Target.Y"=w28, "size"=75.0, "Target.X"=w27, "Bounding Rectangle"=T12 {"Left"=0, "Top"=0, "Right"=0, "Bottom"=0}, "image in"=w21) -> ("image out"=w20:T1)  [unwired: 5 in]
    n13 = case shown="\"\", \"Idle\"" w39 {
      selector: w39 -> [_ _ w162 _ _ _ _ _ _ _ _ _ _ _ _ _ _ _ _ _ _ _ _ _ _ _ _ _ _ _ _ _]
      tunnel: w38 -> [w47 w161 w166 w184 w190 w195 w199 w218 w224 w228 w232 w238 w249 w275 w280 w290 w294 w300 w306 w321 w333 w349 w356 w360 w387 w393 w430 w443 w488 w528 w565 w569]
      tunnel: w37 -> [_ _ _ _ _ _ _ _ _ _ _ w233 w243 _ _ _ _ _ _ _ _ _ _ _ _ _ _ _ _ _ _ _]
      tunnel: w32 -> [w45 w158 w164 w175 w187 w193 w196 _ w220 w225 w230 w236 w245 w272 w277 w287 w291 w296 w302 w317 w329 w340 w352 w357 w367 w395 w427 w433 w479 w525 w557 w566]
      tunnel: [w44 w159 w168 w181 errorcluster {"status"=FALSE, "code"=0, "source"=""} ("error out") w192 w197 w215 w221 w226 w229 w234 w246 w273 w278 w288 w292 w298 w304 w308 w324 w337 w354 w358 w385 w414 w428 w441 w486 w526 w563 w567] -> w35
      tunnel: w30 -> [w43 w159 w167 w181 w186 w192 w197 w215 w222 w226 w229 w235 w247 w273 w278 w288 w292 w298 w304 w309 w325 w338 w354 w358 w385 w414 w428 w441 w486 w526 w563 w567]
      tunnel: [w46 w160 w165 w183 w189 w194 w198 w217 w223 w227 w231 w237 w248 w274 w279 w289 w293 w299 w305 w320 w332 w348 w355 w359 w386 w401 w429 w442 w487 w527 w564 w568] -> w34
      tunnel: [_ _ _ _ _ TRUE _ _ _ _ _ _ _ _ _ _ _ _ _ _ _ _ _ _ _ _ _ _ _ _ _ _] -> w29
      tunnel: [w42 w158 w164 w182 w187 w193 w196 w216 w220 w225 w230 w236 w245 w272 w277 w287 w291 w295 w301 w317 w329 w339 w351 w357 w366 w399 w427 w435 w478 w523 w546 w566] -> w33
      tunnel: "update speed [ms]" -> [w41 _ _ _ _ _ _ _ _ _ _ _ _ _ _ _ _ _ _ _ _ _ _ _ _ _ _ _ _ _ _ _]
      tunnel: w20 -> [w40 _ _ _ _ _ _ _ _ _ _ _ _ _ _ _ _ _ _ _ _ _ _ _ _ _ _ _ _ _ _ _]
      frame "", "Idle" {
        # "executes when the state queue is empty"
        n14 = event shown="[0] Timeout" {
          selector: _ -> [_ _ _ _ _ _ _ _ _ _]
          dyn-events: _ -> [_ _ _ _ _ _ _ _ _ _]
          timeout: w41 -> [_ _ _ _ _ _ _ _ _ _]
          tunnel: w47 -> [w69 w109 w114 w119 w124 w128 w133 w140 w151 w157]
          tunnel: [w68 w108 w112 w117 w122 w127 w132 w140 w150 w156] -> w46
          tunnel: w45 -> [w59 w110 w115 w120 w125 w130 w135 w139 w148 w154]
          tunnel: [w65 w107 w111 w116 w121 w129 w134 w141 w149 w155] -> w44
          tunnel: w43 -> [w84 w107 w111 w116 w121 w129 w134 w141 w149 w155]
          tunnel: [w87 w110 w115 w120 w125 w130 w135 w139 w148 w154] -> w42
          tunnel: w40 -> [w88 _ _ _ _ _ _ _ _ _]
          event Timeout {
            w57 = FALSE ("moving")
            w76 = u32 65421 ("Color")
            n15 = event-data() -> ()  [unwired: 1 in, 1 out]
            n16 = Unbundle By Name(w59) -> ("beam detection para"=w89:T2, "Centriod X"=w86:dbl[], "Centriod Y"=w85:dbl[], "Best Rectangle"=w78:T7)
            n17 = Bundle By Name(cluster=w59, "moving"=w57) -> (w58:T17)
            n18 = local write "moving"(w57) -> ()
            n19 = call "CENTRIOD DETECTION BEAMPOINTING.vi"("Refnum in"=w88, "beam detection para"=w89, "error in (no error)"=w84) -> ("Bounding Rect"=w48:T18, "Particle Reports (Pixels)"=w62:T5, "Refnum out"=w73:T1, "Centriod"=w49:cluster{"X":dbl, "Y":dbl}, "error out"=w67:errorcluster)  [unwired: 10 in, 2 out]
            "Particle Reports (Pixels)" <- w62
            n20 = Unbundle By Name(w49) -> ("X"=w81:dbl, "Y"=w80:dbl)
            n21 = Not Equal To 0?(x=w80) -> (x != 0?=w83:bool)
            n22 = Not Equal To 0?(x=w81) -> (x != 0?=w82:bool)
            n23 = Or(x=w82, y=w83) -> (x .or. y?=w79:bool)
            n24 = case shown="True" w79 {
              tunnel: w86 -> [w96 w105]
              tunnel: w85 -> [w95 w104]
              tunnel: [w96 w103] -> w71
              tunnel: [w95 w102] -> w72
              tunnel: w81 -> [_ w101]
              tunnel: w80 -> [_ w100]
              tunnel: w78 -> [w94 w99]
              tunnel: w48 -> [_ w98]
              tunnel: [w94 w97] -> w77
              frame False {
              }
              frame True {
                n25 = Build Array (concatenate)(w99, w98) -> (w97:T7)
                n26 = Build Array (concatenate)(w104, w100) -> (w102:dbl[])
                n27 = Build Array (concatenate)(w105, w101) -> (w103:dbl[])
              }
            }
            "centriod X" <- w71
            "centriod Y" <- w72
            n28 = call "IMAQ Overlay Rectangle"("Color"=w76, "error in (no error)"=w67, "Rectangle"=w48, "Image"=w73) -> ("error out"=w74:errorcluster, "Image Out"=w75:T1)  [unwired: 6 in]
            n29 = local read "Target.X::1"() -> (w51:dbl)
            n30 = local read "Target.Y::1"() -> (w50:dbl)
            n31 = call "IMAQ Overlay Points"("Color"=w76, "error in (no error)"=w74, "Point"=w49, "Image"=w75) -> ("error out"=w66:errorcluster, "Image Out"=w53:T1)  [unwired: 6 in]
            n32 = local read "img to avg"() -> (w63:i32)
            n33 = Array Size(array=w71) -> (size(s)=w64:i32)
            n34 = call "draw crosshair imaq.vi"("Color"=u32 16774656, "Target.Y"=w50, "size"="size", "Target.X"=w51, "Bounding Rectangle"=T12 {"Left"=0, "Top"=0, "Right"=0, "Bottom"=0}, "image in"=w53) -> ("image out"=→"Beam":T1)  [unwired: 5 in]
            n35 = Greater Or Equal?(x=w64, y=w63) -> (x >= y?=w70:bool)
            n36 = case shown="True" w70 {
              tunnel: w69 -> [w90 w93]
              tunnel: [w90 w92] -> w68
              frame False {
              }
              frame True {
                n37 = call <vilib>:"Add State(s) to Queue__jki_lib_state_machine.vi"("State(s) in (\"\")"=w93, "State(s) at Back (\"\")"="detected" ("State(s) in Front (\"\")")) -> ("States Out"=w92:string)  [unwired: 13 in]
              }
            }
            n38 = Empty Array?(array=w62) -> (empty?=w61:bool)
            n39 = Not(x=w61) -> (.not. x?=w60:bool)
            "beam detected" <- w60
            n40 = Bundle By Name(cluster=w58, "PArticle Report"=w62, "Centriod X"=w71, "Centriod Y"=w72, "Best Rectangle"=w77, "beam detected"=w60) -> (w87:T17)
            n41 = call <vilib>:"Clear Errors.vi"("error in (no error)"=w66) -> ("error out"=w65:errorcluster)  [unwired: 6 in]
          }
          event Value Change {
            n42 = event-data() -> ()  [unwired: 1 in, 6 out]
            n43 = call <vilib>:"Add State(s) to Queue__jki_lib_state_machine.vi"("State(s) in (\"\")"=w109, "State(s) at Back (\"\")"="Beam Detection" ("State(s) at Back (\"\")")) -> ("States Out"=w108:string)  [unwired: 13 in]
          }
          event Value Change {
            n44 = event-data() -> ()  [unwired: 1 in, 6 out]
            n45 = call <vilib>:"Add State(s) to Queue__jki_lib_state_machine.vi"("State(s) in (\"\")"=w114, "State(s) at Back (\"\")"=" Move Properties" ("State(s) at Back (\"\")")) -> ("States Out"=w112:string)  [unwired: 13 in]
          }
          event "Save Config": Value Change {
            n46 = event-data() -> ()  [unwired: 1 in, 6 out]
            n47 = call <vilib>:"Add State(s) to Queue__jki_lib_state_machine.vi"("State(s) in (\"\")"=w119, "State(s) at Back (\"\")"="Save Configuration" ("State(s) in Front (\"\")")) -> ("States Out"=w117:string)  [unwired: 13 in]
          }
          event "Save Stats": Value Change {
            n48 = event-data() -> ()  [unwired: 1 in, 6 out]
            n49 = call <vilib>:"Add State(s) to Queue__jki_lib_state_machine.vi"("State(s) in (\"\")"=w124, "State(s) at Back (\"\")"="Save Stats" ("State(s) in Front (\"\")")) -> ("States Out"=w122:string)  [unwired: 13 in]
          }
          event "Load Config": Value Change {
            n50 = event-data() -> ()  [unwired: 1 in, 6 out]
            n51 = call <vilib>:"Add State(s) to Queue__jki_lib_state_machine.vi"("State(s) in (\"\")"=w128, "State(s) at Back (\"\")"="Load Configuration" ("State(s) in Front (\"\")")) -> ("States Out"=w127:string)  [unwired: 13 in]
          }
          event "Reset History": Value Change {
            n52 = event-data() -> ()  [unwired: 1 in, 6 out]
            n53 = call <vilib>:"Add State(s) to Queue__jki_lib_state_machine.vi"("State(s) in (\"\")"=w133, "State(s) at Back (\"\")"="Reset History" ("State(s) in Front (\"\")")) -> ("States Out"=w132:string)  [unwired: 13 in]
          }
          event "Set Centriod Target": Value Change {
            n54 = event-data() -> ()  [unwired: 1 in, 6 out]
            n55 = Two Button Dialog(message="Do want to update the target?") -> (T button?=w136:bool)  [unwired: 2 in]
            n56 = case shown="True" w136 {
              tunnel: w139 -> [_ w146]
              frame False {
              }
              frame True {
                n57 = Unbundle By Name(w146) -> ("Centriod X"=w145:dbl[], "Centriod Y"=w143:dbl[])
                n58 = Index Array(array=w145) -> (element=w144:dbl)  [unwired: 1 in]
                n59 = Index Array(array=w143) -> (element=w142:dbl)  [unwired: 1 in]
                n60 = property on="Target.Y::1" class="DigNum (strict)"("Val(Sgnl)"=w142) -> ()  [unwired: 2 in, 2 out]
                n61 = property on="Target.X::1" class="DigNum (strict)"("Val(Sgnl)"=w144) -> ()  [unwired: 2 in, 2 out]
              }
            }
            n62 = local write "Set Centriod Target"(FALSE ("Set Centriod Target")) -> ()
          }
          event "stop": Value Change {
            # "Exit Button Value Change (pressed) Event\n(this executes Macro: Exit to terminate the VI)"
            n63 = event-data() -> ()  [unwired: 1 in, 6 out]
            n64 = call <vilib>:"Add State(s) to Queue__jki_lib_state_machine.vi"("State(s) in Front (\"\")"="Macro: Exit", "State(s) in (\"\")"=w151) -> ("States Out"=w150:string)  [unwired: 13 in]
          }
          event Panel Close? {
            # "Discard the event because we'll close the front panel ourselves in Macro: Exit"
            # "Close Panel button (pressed) Event\n(this executes Macro: Exit to terminate the VI)"
            n65 = event-data() -> ()  [unwired: 1 in, 1 out]
            n66 = call <vilib>:"Add State(s) to Queue__jki_lib_state_machine.vi"("State(s) in Front (\"\")"="Macro: Exit", "State(s) in (\"\")"=w157) -> ("States Out"=w156:string)  [unwired: 13 in]
            n67 = event-data("Discard?"=TRUE) -> ()  [unwired: 1 in, 1 out]
          }
        }
      }
      frame "---------- Core ----------" {
        # "Do not put any code in this frame.\n(it is a separator no-op)"
        n68 = call <vilib>:"Add State(s) to Queue__jki_lib_state_machine.vi"("State(s) in (\"\")"=w161) -> ("States Out"=w160:string)  [unwired: 14 in]
      }
      frame Default {
        w171 = 42 items=["No error", "Argument error", "Memory is full", "Out of zone", "End of file", "File already open", "Generic file I/O error", "File not found", "File permission error", "Disk is full", "Duplicate path", "Too many files open", "System feature not enabled", "Resource file not found", "Cannot add resource", "Resource not found", "Image not found", "Image memory error", "Pen does not exist", "Config type invalid", "Config token not found", "Config parse error", "Config memory error", "Bad external code format", "Bad external code offset", "External code not present", "Null window", "Destroy window error", "Null menu", "Print aborted", "Bad print record", "Print driver error", "Windows error during printing", "Memory error during printing", "Print dialog error", "Generic print error", "Invalid device refnum", "Device not found", "Device parameter error", "Device unit error", "Cannot open device", "Device call aborted", "Generic error", "Cancelled by user", "Object ID too low", "Object ID too high", "Object not in heap", "Unknown heap", "Unknown object (invalid DefProc)", "Unknown object (DefProc not in table)", "Message out of range", "Invalid (null) method", "Unknown message", "Manager call not supported", "Bad address", "Network operation in progress", "Network operation timed out", "Connection is busy", "Network attribute not supported", "Network error", "Address in use", "System out of memory", "Connection aborted", "Connection refused", "Not connected", "Already connected", "Connection closed", "Initialization error (interapplication manager)", "Bad occurrence", "Wait on unbound occurrence handler", "Occurrence queue overflow", "Datalog type conflict", "Unused", "Unrecognized type (interapplication manager)", "Memory corrupt", "Failed to make temporary DLL", "Old CIN version", "Drag socket not found", "Failed to load drop-object", "Failed to register OLE object", "Failed to release OLE object", "Format specifier type mismatch", "Unknown format specifier", "Too few format specifiers", "Too many format specifiers", "Scan failed", "Newer CIN version", "Error converting to variant", "Runtime menu error", "Password tampered", "Variant attribute not found", "Incompatible variant data type", "Event data is not available", "Event Store is not present", "Occurrence is not found", "Event Queue is not created", "Event info is not available", "Refnum passed is NULL", "Error retrieving Class GUID", "Error retrieving CoClass GUID", "Error retrieving TypeLib GUID.", "Bad built application magic bytes.", "Specific driver is different from the specific driver associated with the Logical Name.", "There is no session opened to the class driver.", "Max Error", "MAX - Error with config objects", "MAX - Error loading configuration", "MAX - Group not supported"]
        # "Current State"
        # "Do not delete, rename, or modify this frame.\n(this is used to capture unhandled states and typos)"
        # "Handle mistyped state name (developer tool)"
        n69 = Format Into String(format string="Software Exception: Unhandled State \"%s\"." ("message"), error in=w167, w162) -> (resulting string=w170:string, error out=w169:errorcluster)  [unwired: 1 in]
        n70 = call <vilib>:"Error Cluster From Error Code.vi"("show call chain? (False)"=TRUE, "error in (no error)"=w169, "error message (\"\")"=w170, "error code (0)"=w171) -> ("error out"=w168:errorcluster)  [unwired: 5 in]
        n71 = call <vilib>:"Add State(s) to Queue__jki_lib_state_machine.vi"("State(s) in (\"\")"=w166) -> ("States Out"=w165:string)  [unwired: 14 in]
      }
      frame "Initialize Core Data" {
        # "Do not delete, rename, or modify this frame.\n(this is used to determine panel behavior on exit)"
        # "originally closed?"
        # "exe?"
        # "If panel starts closed or is an EXE, then close it when we exit"
        n72 = property class="VI"() -> ("Front Panel.Open"=w180:bool)  [unwired: 2 in, 2 out]
        n73 = property class="App"() -> ("App.Kind"=w179:T13)  [unwired: 2 in, 2 out]
        n74 = control-ref of="Current VI Reference"() -> (w173:refnum<vi>)
        n75 = Not(x=w180) -> (.not. x?=w177:bool)
        n76 = Equal?(x=w179, y=T13."Run Time System" ("Application:Kind")) -> (x = y?=w176:bool)
        n77 = Or(x=w177, y=w176) -> (x .or. y?=w174:bool)
        n78 = Bundle By Name(cluster=w175, "Core.Current VI Reference"=w173, "Core.Close Panel on Exit?"=w174) -> (w182:T17)
        n79 = call <vilib>:"Add State(s) to Queue__jki_lib_state_machine.vi"("State(s) in (\"\")"=w184) -> ("States Out"=w183:string)  [unwired: 14 in]
      }
      frame "Error Handler" {
        # "Unhandled Error -- Display it"
        # "Handle any errors here.\nYou can also output any states to clean-up after errors occur"
        # "Clear error"
        n80 = call <vilib>:"General Error Handler.vi"("error in (no error)"=w186) -> ()  [unwired: 10 in, 5 out]
        n81 = call <vilib>:"Add State(s) to Queue__jki_lib_state_machine.vi"("State(s) in Front (\"\")"="/* Post Error States", "State(s) in (\"\")"=w190) -> ("States Out"=w189:string)  [unwired: 13 in]
      }
      frame "Exit" {
        # "Do not put any code in this frame.\n(No errors that occur here will be handled.)"
        n82 = call <vilib>:"Add State(s) to Queue__jki_lib_state_machine.vi"("State(s) in (\"\")"=w195) -> ("States Out"=w194:string)  [unwired: 14 in]
      }
      frame "---------- Data ----------" {
        # "Do not put any code in this frame.\n(It is a separator no-op. You can make a copy of this frame to create a new Data frame)"
        n83 = call <vilib>:"Add State(s) to Queue__jki_lib_state_machine.vi"("State(s) in (\"\")"=w199) -> ("States Out"=w198:string)  [unwired: 14 in]
      }
      frame "Data: Initialize" {
        w200 = FALSE  # set centriod target
        w201 = T16 {"Stat Centriod X"=[], "Stat Centriod Y"=[], "TRA Position X"=[], "TRA PositionY"=[], "Time"=[]}  # Stats
        w204 = FALSE  # moving
        w203 = T4 {"Tolerance [%]"=10.0, "Stepsize"=0.0, "Invert Axis"=FALSE, "Invert Direction X"=FALSE, "Invert Direction Y"=FALSE, "enable feedback"=FALSE}  # move
        w205 = cluster{"X offset":dbl, "Y offset":dbl} {"X offset"=0.0, "Y offset"=0.0}  # offsets
        w206 = FALSE  # beam detected
        w202 = T2 {"Filter"=1, "Filter Para"={"X Size"=5, "Y Size"=5, "% Tolerance"=1}, "detection method"=4, "smal para"=[{"Measurement Parameter"=35, "Range Lower Value"=0.0, "Range Upper Value"=500.0, "Range"=TRUE, "Measurement Type"=FALSE}], "Remove small Objects"=TRUE, "Restrict to round Objects"=FALSE}  # beam detection para
        w207 = timestamp[] []  # Time
        w208 = dbl[] []  # Mean Centriod Y
        w209 = dbl[] []  # Mean Centriod X
        w210 = T5 [{"Area"=1104.0, "Number of Holes"=0.0, "Bounding Rect"={"Left"=378.0, "Top"=230.0, "Right"=422.0, "Bottom"=264.0}, "Center of Mass"={"X"=399.60235507246375, "Y"=246.169384057971}, "Orientation"=6.346766143267859, "Dimensions"={"Width"=44.0, "Height"=34.0}}]  # PArticle Report
        w211 = T7 []  # Best Rectangle
        w212 = dbl[] []  # Centriod Y
        w213 = dbl[] []  # Centriod X
        w214 = T19 {"Current VI Reference"=refnum, "Close Panel on Exit?"=FALSE}  # Core
        # "Initialize the shift-register data, here.\n(data names are defined by what you wire into the bundle function)"
        n84 = local write "beam detection para"(w202) -> ()
        n85 = Bundle("Core"=w214, "beam detection para"=w202, "Centriod X"=w213, "Centriod Y"=w212, "Best Rectangle"=w211, "PArticle Report"=w210, "Mean Centriod X"=w209, "Mean Centriod Y"=w208, "Time"=w207, "beam detected"=w206, "offsets"=w205, "move"=w203, "moving"=w204, "Stats"=w201, "set centriod target"=w200) -> (w216:T17)  [unwired: 1 in]
        n86 = call <vilib>:"Add State(s) to Queue__jki_lib_state_machine.vi"("State(s) in (\"\")"=w218) -> ("States Out"=w217:string)  [unwired: 14 in]
        n87 = local write "Move Properties"(w203) -> ()
      }
      frame "Data: Cleanup" {
        # "Cleanup any data and references, here.\n(this is called automatically, by the Macro: Exit)"
        n88 = Unbundle By Name(w220) -> ("Core.Current VI Reference"=w219:refnum<vi>)
        n89 = Close Reference(reference=w219, error in (no error)=w222) -> (error out=w221:errorcluster)
        n90 = call <vilib>:"Add State(s) to Queue__jki_lib_state_machine.vi"("State(s) in (\"\")"=w224) -> ("States Out"=w223:string)  [unwired: 14 in]
      }
      frame "---------- UI ----------" {
        # "Do not put any code in this frame.\n(It is a separator no-op. You can make a copy of this frame to create a new UI frame)"
        n91 = call <vilib>:"Add State(s) to Queue__jki_lib_state_machine.vi"("State(s) in (\"\")"=w228) -> ("States Out"=w227:string)  [unwired: 14 in]
      }
      frame "UI: Initialize" {
        # "Initialize the User Interface, here.\n(this is called automatically, by the Macro: Init)"
        n92 = call <vilib>:"Add State(s) to Queue__jki_lib_state_machine.vi"("State(s) in (\"\")"=w232) -> ("States Out"=w231:string)  [unwired: 14 in]
      }
      frame "UI: Cursor Set" {
        # "Argument"
        # "Set and Unset Cursor Busy.\n(Usage: \"UI: Cursor Set >> Busy|Idle\")"
        n93 = case shown="\"Idle\", Default" w233 {
          tunnel: w235 -> [w240 w242]
          tunnel: [w239 w241] -> w234
          frame "Idle", Default {
            n94 = call <vilib>:"Unset Busy.vi"("error in (no error)"=w240) -> ("error out"=w239:errorcluster)  [unwired: 10 in]
          }
          frame "Busy" {
            n95 = call <vilib>:"Set Busy.vi"("error in (no error)"=w242) -> ("error out"=w241:errorcluster)  [unwired: 9 in, 1 out]
          }
        }
        n96 = call <vilib>:"Add State(s) to Queue__jki_lib_state_machine.vi"("State(s) in (\"\")"=w238) -> ("States Out"=w237:string)  [unwired: 14 in]
      }
      frame "UI: Front Panel State" {
        # "Argument"
        # "Set Front Panel Open or Closed\n(Usage: \"UI: Front Panel State >> Open|Close\")"
        n97 = Unbundle By Name(w245) -> ("Core.Current VI Reference"=w244:refnum<vi>)
        n98 = case shown="\"Close\"" w243 {
          tunnel: w247 -> [w253 w266]
          tunnel: [w255 w267] -> w246
          tunnel: w244 -> [w254 w264]
          frame "Open", Default {
            n99 = property class="VI"(reference=w254, error in=w253) -> (reference out=w251:refnum<vi>, error out=w252:errorcluster, "Front Panel.Open"=w250:bool)
            n100 = case shown="False" w250 {
              tunnel: [w258 w261] -> w255
              tunnel: w252 -> [w257 w261]
              tunnel: w251 -> [w256 _]
              frame False {
                n101 = invoke class="VI" method="FP.Open"(reference=w256, error in=w257, "Activate"=TRUE, "State"=T14."Standard") -> (error out=w258:errorcluster)  [unwired: 1 in, 4 out]
              }
              frame True {
              }
            }
          }
          frame "Close" {
            n102 = property class="VI"(reference=w264, error in=w266) -> (reference out=w263:refnum<vi>, error out=w265:errorcluster, "Front Panel.Open"=w262:bool)
            n103 = case shown="True" w262 {
              tunnel: [w268 w271] -> w267
              tunnel: w265 -> [w268 w270]
              tunnel: w263 -> [_ w269]
              frame False {
              }
              frame True {
                n104 = invoke class="VI" method="FP.Close"(reference=w269, error in=w270) -> (error out=w271:errorcluster)  [unwired: 1 in, 2 out]
              }
            }
          }
        }
        n105 = call <vilib>:"Add State(s) to Queue__jki_lib_state_machine.vi"("State(s) in (\"\")"=w249) -> ("States Out"=w248:string)  [unwired: 14 in]
      }
      frame "---------- Macro ----------" {
        # "Do not put any code in this frame.\n(It is a separator no-op. You can make a copy of this frame to create a new Macro frame)"
        n106 = call <vilib>:"Add State(s) to Queue__jki_lib_state_machine.vi"("State(s) in (\"\")"=w275) -> ("States Out"=w274:string)  [unwired: 14 in]
      }
      frame "Macro: Initialize" {
        w276 = "Data: Initialize\nInitialize Core Data\nUI: Initialize\nUI: Front Panel State >> Open"  # Data: Initialize Initialize Core Data UI: Initialize UI: Front Panel State >> Open
        # "Initialization Macro\n(This is called once, when the VI starts)"
        n107 = call <vilib>:"Add State(s) to Queue__jki_lib_state_machine.vi"("State(s) in Front (\"\")"=w276, "State(s) in (\"\")"=w280) -> ("States Out"=w279:string)  [unwired: 13 in]
      }
      frame "Macro: Exit" {
        # "Exit Macro\n(This is called once, when the VI exits)"
        n108 = Unbundle By Name(w287) -> ("Core.Close Panel on Exit?"=w285:bool)
        n109 = Select(t="UI: Front Panel State >> Close", s=w285, f="") -> (s? t:f=w282:string)
        n110 = call <vilib>:"Add State(s) to Queue__jki_lib_state_machine.vi"("State(s) in (\"\")"=w282, "State(s) at Back (\"\")"="Data: Cleanup\nExit") -> ("States Out"=w286:string)  [unwired: 13 in]
        n111 = call <vilib>:"Add State(s) to Queue__jki_lib_state_machine.vi"("State(s) in Front (\"\")"=w286, "State(s) in (\"\")"=w290) -> ("States Out"=w289:string)  [unwired: 13 in]
      }
      frame "-------------Properties---------" {
        # "Template Separator\n(You can make a copy of, or modify, this frame)"
        n112 = call <vilib>:"Add State(s) to Queue__jki_lib_state_machine.vi"("State(s) in (\"\")"=w294) -> ("States Out"=w293:string)  [unwired: 14 in]
      }
      frame "Beam Detection" {
        # "Your code here.\n(You can make a copy of, or modify, this frame)"
        n113 = Bundle By Name(cluster=w296, "beam detection para"="beam detection para") -> (w295:T17)
        n114 = call <vilib>:"Add State(s) to Queue__jki_lib_state_machine.vi"("State(s) in (\"\")"=w300) -> ("States Out"=w299:string)  [unwired: 14 in]
      }
      frame "Move Properties" {
        n115 = Bundle By Name(cluster=w302, "move"="Move Properties") -> (w301:T17)
        n116 = call <vilib>:"Add State(s) to Queue__jki_lib_state_machine.vi"("State(s) in (\"\")"=w306) -> ("States Out"=w305:string)  [unwired: 14 in]
      }
      frame "Save Configuration" {
        n117 = Unbundle By Name(w317) -> ("beam detection para"=w315:T2, "move"=w314:T4)
        n118 = local read "img to avg"() -> (w316:i32)
        n119 = Bundle("img to avg"=w316, "beam detection para"=w315, "move"=w314) -> (w313:T6)  [unwired: 1 in]
        n120 = Open/Create/Replace File(error in=w309, operation (0:open)=T15."replace or create with confirmation") -> (refnum out=w318:refnum<file>, error out=w312:errorcluster)  [unwired: 4 in, 1 out]
        n121 = Write to Binary File(file (use dialog)=w318, data=w313, error in=w312) -> (refnum out=w310:refnum<file>, error out=w311:errorcluster)  [unwired: 3 in, 1 out]
        n122 = Close File(refnum=w310, error in=w311) -> (error out=w308:errorcluster)  [unwired: 1 out]
        n123 = local write "Save Config"(FALSE ("Save Button")) -> ()
        n124 = call <vilib>:"Add State(s) to Queue__jki_lib_state_machine.vi"("State(s) in (\"\")"=w321) -> ("States Out"=w320:string)  [unwired: 14 in]
      }
      frame "Save Stats" {
        n125 = Unbundle By Name(w329) -> ("Stats"=w322:T16)
        n126 = Open/Create/Replace File(error in=w325, operation (0:open)=T15."replace or create with confirmation") -> (refnum out=w330:refnum<file>, error out=w328:errorcluster)  [unwired: 4 in, 1 out]
        n127 = Write to Binary File(file (use dialog)=w330, data=w322, error in=w328) -> (refnum out=w326:refnum<file>, error out=w327:errorcluster)  [unwired: 3 in, 1 out]
        n128 = Close File(refnum=w326, error in=w327) -> (error out=w324:errorcluster)  [unwired: 1 out]
        n129 = call <vilib>:"Add State(s) to Queue__jki_lib_state_machine.vi"("State(s) in (\"\")"=w333) -> ("States Out"=w332:string)  [unwired: 14 in]
        n130 = local write "Save Stats"(FALSE ("Save Button")) -> ()
      }
      frame "Load Configuration" {
        # "Your code here.\n(You can make a copy of, or modify, this frame)"
        n131 = Open/Create/Replace File(error in=w338, operation (0:open)=T15."open") -> (refnum out=w346:refnum<file>, error out=w345:errorcluster)  [unwired: 4 in, 1 out]
        n132 = Read from Binary File(5:"save cluster", 8:w345, 11:w346) -> (0:w344:errorcluster, 2:w341:T6, 3:w343:refnum<file>)  [unwired: 3 in, 1 out]
        n133 = Close File(refnum=w343, error in=w344) -> (error out=w337:errorcluster)  [unwired: 1 out]
        n134 = Unbundle By Name(w341) -> ("beam detection para"=w336:T2, "move"=w335:T4)  [unwired: 1 out]
        n135 = Bundle By Name(cluster=w340, "beam detection para"=w336, "move"=w335) -> (w339:T17)
        n136 = local write "beam detection para"(w336) -> ()
        n137 = local write "Move Properties"(w335) -> ()
        n138 = call <vilib>:"Add State(s) to Queue__jki_lib_state_machine.vi"("State(s) in (\"\")"=w349) -> ("States Out"=w348:string)  [unwired: 14 in]
        n139 = local write "Load Config"(FALSE ("Load Button")) -> ()
      }
      frame "Reset History" {
        w353 = dbl[] [] ("Mean Centriod X")
        # "Your code here.\n(You can make a copy of, or modify, this frame)"
        n140 = local write "Reset History"(FALSE ("Reset History")) -> ()
        n141 = call <vilib>:"Add State(s) to Queue__jki_lib_state_machine.vi"("State(s) in (\"\")"=w356) -> ("States Out"=w355:string)  [unwired: 14 in]
        n142 = Bundle By Name(cluster=w352, "Mean Centriod X"=w353, "Mean Centriod Y"=w353) -> (w351:T17)
      }
      frame "---------- centriod analysis----------" {
        # "Template Separator\n(You can make a copy of, or modify, this frame)"
        n143 = call <vilib>:"Add State(s) to Queue__jki_lib_state_machine.vi"("State(s) in (\"\")"=w360) -> ("States Out"=w359:string)  [unwired: 14 in]
      }
      frame "detected" {
        w384 = dbl[] [] ("Array")
        n144 = Unbundle By Name(w367) -> ("Time"=w377:timestamp[], "Centriod X"=w372:dbl[], "Mean Centriod X"=w376:dbl[], "Centriod Y"=w371:dbl[], "Mean Centriod Y"=w375:dbl[], "Best Rectangle"=→"Best Rectangle":T7)
        n145 = local read "Target.X::1"() -> (w374:dbl)
        n146 = local read "Target.Y::1"() -> (w373:dbl)
        n147 = call <vilib>:"Std Deviation and Variance.vi"("X"=w372) -> ("mean"=w378:dbl)  [unwired: 1 in, 2 out]
        "mean X" <- w378
        n148 = call <vilib>:"Std Deviation and Variance.vi"("X"=w371) -> ("mean"=w379:dbl)  [unwired: 1 in, 2 out]
        "mean Y" <- w379
        n149 = Subtract(x=w374, y=w378) -> (x-y=w365:dbl)
        "X offset" <- w365
        n150 = Subtract(x=w373, y=w379) -> (x-y=w364:dbl)
        "Y offset" <- w364
        n151 = Get Date/Time In Seconds() -> (seconds since 1Jan1904=w380:timestamp)
        n152 = Build Array (concatenate)(w376, w365) -> (w369:dbl[])
        n153 = Build Array (concatenate)(w375, w364) -> (w368:dbl[])
        n154 = Build Array (concatenate)(w377, w380) -> (w370:timestamp[])
        n155 = Bundle(w365, w364) -> (w363:cluster{dbl, dbl})  [unwired: 1 in]
        n156 = Bundle(w370, w369) -> (w381:cluster{timestamp[], dbl[]})  [unwired: 1 in]
        n157 = Bundle(w370, w368) -> (w382:cluster{timestamp[], dbl[]})  [unwired: 1 in]
        n158 = call <vilib>:"Add State(s) to Queue__jki_lib_state_machine.vi"("State(s) in (\"\")"=w387, "State(s) at Back (\"\")"="check move") -> ("States Out"=w386:string)  [unwired: 13 in]
        n159 = Build Array(w381, w382) -> (→"XY Graph":cluster{timestamp[], dbl[]}[])
        n160 = Bundle By Name(cluster=w367, "Time"=w370, "Mean Centriod X"=w369, "Mean Centriod Y"=w368, "Centriod X"=w384, "Centriod Y"=w384, "offsets"=w363) -> (w366:T17)
      }
      frame "check move" {
        n161 = Unbundle By Name(w395) -> ("Best Rectangle"=w413:T7, "offsets.X offset"=w412:dbl, "offsets.Y offset"=w411:dbl)
        n162 = Absolute Value(x=w412) -> (abs(x)=w408:dbl)
        n163 = Absolute Value(x=w411) -> (abs(x)=w405:dbl)
        n164 = Unbundle By Name(w395) -> ("move.Tolerance [%]"=w410:dbl)
        n165 = call "Beam Size.vi"("Best Rectangle"=w413) -> ("Y Size"=w391:dbl, "X Size"=w392:dbl)  [unwired: 9 in]
        "X Size" <- w392
        "Y Size" <- w391
        n166 = Divide(x=w410, y=100.0) -> (x/y=w406:dbl)
        n167 = Multiply(x=w406, y=w392) -> (x*y=w407:dbl)
        n168 = Multiply(x=w406, y=w391) -> (x*y=w404:dbl)
        n169 = Max & Min(x=w392, y=w391) -> (max(x,y)=w390:dbl)  [unwired: 1 out]
        n170 = Divide(x=w390, y=2.0) -> (x/y=w388:dbl)
        n171 = Greater Or Equal?(x=w408, y=w407) -> (x >= y?=w398:bool)
        n172 = Greater Or Equal?(x=w405, y=w404) -> (x >= y?=w397:bool)
        n173 = local write "size"(w388) -> ()
        n174 = case shown="True" w397 {
          tunnel: w393 -> [w419 w422]
          tunnel: [w419 w420] -> w403
          frame False {
          }
          frame True {
            n175 = call <vilib>:"Add State(s) to Queue__jki_lib_state_machine.vi"("State(s) in (\"\")"=w422, "State(s) at Back (\"\")"="Move Y" ("State(s) at Back (\"\")")) -> ("States Out"=w420:string)  [unwired: 13 in]
          }
        }
        n176 = case shown="True" w398 {
          tunnel: w393 -> [w423 w426]
          tunnel: [w423 w424] -> w402
          frame False {
          }
          frame True {
            n177 = call <vilib>:"Add State(s) to Queue__jki_lib_state_machine.vi"("State(s) in (\"\")"=w426, "State(s) at Back (\"\")"="Move X" ("State(s) at Back (\"\")")) -> ("States Out"=w424:string)  [unwired: 13 in]
          }
        }
        n178 = Or(x=w398, y=w397) -> (x .or. y?=w396:bool)
        n179 = Unbundle By Name(w395) -> ("move.enable feedback"=w394:bool)
        n180 = local write "move required"(w396) -> ()
        n181 = Bundle By Name(cluster=w395, "Best Rectangle"=T7 []) -> (w399:T17)
        n182 = case shown="True" w394 {
          tunnel: w403 -> [_ w418]
          tunnel: w402 -> [_ w417]
          tunnel: [w415 w416] -> w401
          tunnel: w393 -> [w415 _]
          frame False {
          }
          frame True {
            n183 = call <vilib>:"Add State(s) to Queue__jki_lib_state_machine.vi"("State(s) in (\"\")"=w417, "State(s) at Back (\"\")"=w418) -> ("States Out"=w416:string)  [unwired: 13 in]
          }
        }
      }
      frame "-----------Motor Move---------" {
        # "Your code here.\n(You can make a copy of, or modify, this frame)"
        n184 = call <vilib>:"Add State(s) to Queue__jki_lib_state_machine.vi"("State(s) in (\"\")"=w430) -> ("States Out"=w429:string)  [unwired: 14 in]
      }
      frame "Move X" {
        w434 = TRUE ("moving")
        n185 = Unbundle By Name(w433) -> ("move.Invert Direction X"=w440:bool, "move.Invert Axis"=w438:bool, "move.Stepsize"=w439:dbl, "offsets.X offset"=w432:dbl)
        "move.Stepsize" <- w439
        n186 = Greater Than 0?(x=w432) -> (x > 0?=w431:bool)
        n187 = Unbundle By Name(w433) -> ("move.Invert Axis"=w437:bool)
        n188 = case shown="False" w431 {
          tunnel: w440 -> [w449 w465]
          tunnel: w439 -> [w447 w463]
          tunnel: w438 -> [w446 w462]
          tunnel: w437 -> [w445 w461]
          frame True {
            n189 = case shown="True" w446 {
              tunnel: [w458 w459] -> w448
              frame False {
                n190 = local read "Position.Axis 1::2"() -> (w458:dbl)
              }
              frame True {
                n191 = local read "Position.Axis 2::2"() -> (w459:dbl)
              }
            }
            n192 = case shown="True" w449 {
              tunnel: w448 -> [w454 w457]
              tunnel: w447 -> [w453 w456]
              tunnel: [w452 w455] -> w444
              frame False {
                n193 = Add(x=w454, y=w453) -> (x+y=w452:dbl)
              }
              frame True {
                n194 = Subtract(x=w457, y=w456) -> (x-y=w455:dbl)
              }
            }
            n195 = case shown="True" w445 {
              tunnel: w444 -> [w450 w451]
              frame False {
                n196 = property on="Position.Axis 1::2" class="DigNum (strict)"("Val(Sgnl)"=w450) -> ()  [unwired: 2 in, 2 out]
              }
              frame True {
                n197 = property on="Position.Axis 2::2" class="DigNum (strict)"("Val(Sgnl)"=w451) -> ()  [unwired: 2 in, 2 out]
              }
            }
          }
          frame False {
            n198 = case shown="True" w462 {
              tunnel: [w474 w475] -> w464
              frame False {
                n199 = local read "Position.Axis 1::2"() -> (w474:dbl)
              }
              frame True {
                n200 = local read "Position.Axis 2::2"() -> (w475:dbl)
              }
            }
            n201 = case shown="False" w465 {
              tunnel: w464 -> [w470 w473]
              tunnel: w463 -> [w469 w472]
              tunnel: [w468 w471] -> w460
              frame False {
                n202 = Subtract(x=w470, y=w469) -> (x-y=w468:dbl)
              }
              frame True {
                n203 = Add(x=w473, y=w472) -> (x+y=w471:dbl)
              }
            }
            n204 = case shown="True" w461 {
              tunnel: w460 -> [w466 w467]
              frame False {
                n205 = property on="Position.Axis 1::2" class="DigNum (strict)"("Val(Sgnl)"=w466) -> ()  [unwired: 2 in, 2 out]
              }
              frame True {
                n206 = property on="Position.Axis 2::2" class="DigNum (strict)"("Val(Sgnl)"=w467) -> ()  [unwired: 2 in, 2 out]
              }
            }
          }
        }
        n207 = call <vilib>:"Add State(s) to Queue__jki_lib_state_machine.vi"("State(s) in Front (\"\")"="Wait", "State(s) in (\"\")"=w443) -> ("States Out"=w442:string)  [unwired: 13 in]
        n208 = Bundle By Name(cluster=w433, "moving"=w434) -> (w435:T17)
        n209 = local write "moving"(w434) -> ()
      }
      frame "Move Y" {
        w480 = TRUE ("moving")
        n210 = Unbundle By Name(w479) -> ("move.Invert Direction Y"=w485:bool, "move.Invert Axis"=w483:bool, "move.Stepsize"=w484:dbl, "offsets.Y offset"=w477:dbl)
        "move.Stepsize 2" <- w484
        n211 = Greater Than 0?(x=w477) -> (x > 0?=w476:bool)
        n212 = Unbundle By Name(w479) -> ("move.Invert Axis"=w482:bool)
        n213 = case shown="True" w476 {
          tunnel: w485 -> [w494 w510]
          tunnel: w484 -> [w492 w508]
          tunnel: w483 -> [w491 w507]
          tunnel: w482 -> [w490 w506]
          frame True {
            n214 = case shown="False" w491 {
              tunnel: [w503 w504] -> w493
              frame False {
                n215 = local read "Position.Axis 2::2"() -> (w503:dbl)
              }
              frame True {
                n216 = local read "Position.Axis 1::2"() -> (w504:dbl)
              }
            }
            n217 = case shown="True" w494 {
              tunnel: w493 -> [w499 w502]
              tunnel: w492 -> [w498 w501]
              tunnel: [w497 w500] -> w489
              frame False {
                n218 = Add(x=w499, y=w498) -> (x+y=w497:dbl)
              }
              frame True {
                n219 = Subtract(x=w502, y=w501) -> (x-y=w500:dbl)
              }
            }
            n220 = case shown="True" w490 {
              tunnel: w489 -> [w495 w496]
              frame False {
                n221 = property on="Position.Axis 2::2" class="DigNum (strict)"("Val(Sgnl)"=w495) -> ()  [unwired: 2 in, 2 out]
              }
              frame True {
                n222 = property on="Position.Axis 1::2" class="DigNum (strict)"("Val(Sgnl)"=w496) -> ()  [unwired: 2 in, 2 out]
              }
            }
          }
          frame False {
            n223 = case shown="True" w507 {
              tunnel: [w519 w520] -> w509
              frame False {
                n224 = local read "Position.Axis 2::2"() -> (w519:dbl)
              }
              frame True {
                n225 = local read "Position.Axis 1::2"() -> (w520:dbl)
              }
            }
            n226 = case shown="True" w510 {
              tunnel: w509 -> [w515 w518]
              tunnel: w508 -> [w514 w517]
              tunnel: [w513 w516] -> w505
              frame False {
                n227 = Subtract(x=w515, y=w514) -> (x-y=w513:dbl)
              }
              frame True {
                n228 = Add(x=w518, y=w517) -> (x+y=w516:dbl)
              }
            }
            n229 = case shown="True" w506 {
              tunnel: w505 -> [w511 w512]
              frame False {
                n230 = property on="Position.Axis 2::2" class="DigNum (strict)"("Val(Sgnl)"=w511) -> ()  [unwired: 2 in, 2 out]
              }
              frame True {
                n231 = property on="Position.Axis 1::2" class="DigNum (strict)"("Val(Sgnl)"=w512) -> ()  [unwired: 2 in, 2 out]
              }
            }
          }
        }
        n232 = call <vilib>:"Add State(s) to Queue__jki_lib_state_machine.vi"("State(s) in Front (\"\")"="Wait", "State(s) in (\"\")"=w488) -> ("States Out"=w487:string)  [unwired: 13 in]
        n233 = Bundle By Name(cluster=w479, "moving"=w480) -> (w478:T17)
        n234 = local write "moving"(w480) -> ()
      }
      frame "Wait" {
        w524 = TRUE ("moving")
        # "Wait as long as the motor is moving"
        n235 = while {
          tunnel: w525 -> [w529]
          tunnel: [w529] -> w522
          stop <- w530 stop-if-true
          w533 = StatusTRA_TypDef."MOVING" ("y")
          n236 = local read "Status.Axis 1::2"() -> (w535:T8)
          n237 = local read "Status.Axis 2::2"() -> (w534:T8)
          n238 = Not Equal?(x=w535, y=w533) -> (x != y?=w532:bool)
          n239 = Not Equal?(x=w534, y=w533) -> (x != y?=w531:bool)
          n240 = And(x=w532, y=w531) -> (x .and. y?=w530:bool)
        }
        n241 = Unbundle By Name(w522) -> ()  [unwired: 1 out]
        n242 = call <vilib>:"Add State(s) to Queue__jki_lib_state_machine.vi"("State(s) in (\"\")"=w528, "State(s) at Back (\"\")"="Stats" ("State(s) at Back (\"\")")) -> ("States Out"=w527:string)  [unwired: 13 in]
        n243 = Bundle By Name(cluster=w522, "moving"=w524) -> (w523:T17)
        n244 = local write "moving"(w524) -> ()
      }
      frame "Stats" {
        # "Your code here.\n(You can make a copy of, or modify, this frame)"
        n245 = Unbundle By Name(w557) -> ("Stats.TRA Position X"=w562:dbl[], "Stats.TRA PositionY"=w561:dbl[], "Stats.Stat Centriod X"=w554:dbl[], "Mean Centriod Y"=w553:dbl[], "Stats.Time"=w549:timestamp[])
        n246 = local read "Position.Axis 2::2"() -> (w560:dbl)
        n247 = local read "Position.Axis 1::2"() -> (w559:dbl)
        n248 = local read "Y offset"() -> (w551:dbl)
        n249 = local read "X offset"() -> (w552:dbl)
        n250 = Get Date/Time In Seconds() -> (seconds since 1Jan1904=w548:timestamp)
        n251 = Build Array (concatenate)(w561, w560) -> (w556:dbl[])
        n252 = Build Array (concatenate)(w554, w552) -> (w555:dbl[])
        n253 = Build Array (concatenate)(w553, w551) -> (w550:dbl[])
        n254 = Build Array (concatenate)(w549, w548) -> (w547:timestamp[])
        n255 = Build Array (concatenate)(w562, w559) -> (w558:dbl[])
        n256 = Bundle By Name(cluster=w557, "Stats.TRA Position X"=w558, "Stats.TRA PositionY"=w556, "Stats.Stat Centriod X"=w555, "Stats.Stat Centriod Y"=w550, "Stats.Time"=w547) -> (w546:T17)
        n257 = Unbundle By Name(w546) -> ("Stats.Time"=w542:timestamp[], "Stats.Stat Centriod X"=w545:dbl[], "Stats.Stat Centriod Y"=w544:dbl[], "Stats.TRA Position X"=w543:dbl[], "Stats.TRA PositionY"=w541:dbl[])
        n258 = call <vilib>:"Add State(s) to Queue__jki_lib_state_machine.vi"("State(s) in (\"\")"=w565) -> ("States Out"=w564:string)  [unwired: 14 in]
        n259 = Bundle("Time"=w542, "Stat Centriod X"=w545) -> (w540:T20)  [unwired: 1 in]
        n260 = Bundle("Time"=w542, "Stat Centriod Y"=w544) -> (w539:T21)  [unwired: 1 in]
        n261 = Bundle("Time"=w542, "TRA Position X"=w543) -> (w538:T22)  [unwired: 1 in]
        n262 = Bundle("Time"=w542, "TRA PositionY"=w541) -> (w537:T23)  [unwired: 1 in]
        n263 = Build Array(w540, w539, w538, w537) -> (→"Stats":T24)
      }
      frame "New Category: 2" {
        # "Your code here.\n(You can make a copy of, or modify, this frame)"
        n264 = call <vilib>:"Add State(s) to Queue__jki_lib_state_machine.vi"("State(s) in (\"\")"=w569) -> ("States Out"=w568:string)  [unwired: 14 in]
      }
    }
  }
  n265 = control-ref of="This Application"() -> (w5:refnum<vi>)
  n266 = control-ref of="This VI"() -> (w9:refnum<vi>)
  n267 = Current VI's Menubar() -> (w8:refnum<k9>)
  n268 = call "GUI_Master_subvi_reentrant_queues.vi"("This Application"=w5, "error in (no error)"=w6, "tcp data event"=w4, "Caller menu reference"=w8, "Caller VI ref"=w9) -> ("error out"=w17:errorcluster)  [unwired: 6 in]
  n269 = call <vilib>:"Clear Errors.vi"("error in (no error)"=w17) -> ("error out"=w15:errorcluster)  [unwired: 6 in]
  n270 = call "IMAQ Dispose"("error in (no error)"=w15) -> ("error out"=w14:errorcluster)  [unwired: 5 in]
  n271 = call "IMAQ Dispose"("Image"=w10, "error in (no error)"=w14) -> ("error out"=→"error IO 2":errorcluster)  [unwired: 4 in]
